vi "bg image creation-U16.vi"(0 "Array in":path[](array[path])=[path "G:/ViFFIdata/170721EuglenaN+N-/170721EuglenaN--7/N--7_00001.tif", path "G:/ViFFIdata/170721EuglenaN+N-/170721EuglenaN--7/N--7_00002.tif", path "G:/ViFFIdata/170721EuglenaN+N-/170721EuglenaN--7/N--7_00003.tif", path "G:/ViFFIdata/170721EuglenaN+N-/170721EuglenaN--7/N--7_00004.tif", path "G:/ViFFIdata/170721EuglenaN+N-/170721EuglenaN--7/N--7_00005.tif", path "G:/ViFFIdata/170721EuglenaN+N-/170721EuglenaN--7/N--7_00006.tif", path "G:/ViFFIdata/170721EuglenaN+N-/170721EuglenaN--7/N--7_00007.tif", path "G:/ViFFIdata/170721EuglenaN+N-/170721EuglenaN--7/N--7_00008.tif", path "G:/ViFFIdata/170721EuglenaN+N-/170721EuglenaN--7/N--7_00009.tif", path "G:/ViFFIdata/170721EuglenaN+N-/170721EuglenaN--7/N--7_00010.tif", path "G:/ViFFIdata/170721EuglenaN+N-/170721EuglenaN--7/N--7_00011.tif", path "G:/ViFFIdata/170721EuglenaN+N-/170721EuglenaN--7/N--7_00012.tif", path "G:/ViFFIdata/170721EuglenaN+N-/170721EuglenaN--7/N--7_00013.tif", path "G:/ViFFIdata/170721EuglenaN+N-/170721EuglenaN--7/N--7_00014.tif", path "G:/ViFFIdata/170721EuglenaN+N-/170721EuglenaN--7/N--7_00015.tif", path "G:/ViFFIdata/170721EuglenaN+N-/170721EuglenaN--7/N--7_00016.tif", path "G:/ViFFIdata/170721EuglenaN+N-/170721EuglenaN--7/N--7_00017.tif", path "G:/ViFFIdata/170721EuglenaN+N-/170721EuglenaN--7/N--7_00018.tif", path "G:/ViFFIdata/170721EuglenaN+N-/170721EuglenaN--7/N--7_00019.tif", path "G:/ViFFIdata/170721EuglenaN+N-/170721EuglenaN--7/N--7_00020.tif", path "G:/ViFFIdata/170721EuglenaN+N-/170721EuglenaN--7/N--7_00021.tif", path "G:/ViFFIdata/170721EuglenaN+N-/170721EuglenaN--7/N--7_00022.tif", path "G:/ViFFIdata/170721EuglenaN+N-/170721EuglenaN--7/N--7_00023.tif", path "G:/ViFFIdata/170721EuglenaN+N-/170721EuglenaN--7/N--7_00024.tif", path "G:/ViFFIdata/170721EuglenaN+N-/170721EuglenaN--7/N--7_00025.tif", path "G:/ViFFIdata/170721EuglenaN+N-/170721EuglenaN--7/N--7_00026.tif", path "G:/ViFFIdata/170721EuglenaN+N-/170721EuglenaN--7/N--7_00027.tif", path "G:/ViFFIdata/170721EuglenaN+N-/170721EuglenaN--7/N--7_00028.tif", path "G:/ViFFIdata/170721EuglenaN+N-/170721EuglenaN--7/N--7_00029.tif", path "G:/ViFFIdata/170721EuglenaN+N-/170721EuglenaN--7/N--7_00030.tif", path "G:/ViFFIdata/170721EuglenaN+N-/170721EuglenaN--7/N--7_00031.tif", path "G:/ViFFIdata/170721EuglenaN+N-/170721EuglenaN--7/N--7_00032.tif", path "G:/ViFFIdata/170721EuglenaN+N-/170721EuglenaN--7/N--7_00033.tif", path "G:/ViFFIdata/170721EuglenaN+N-/170721EuglenaN--7/N--7_00034.tif", path "G:/ViFFIdata/170721EuglenaN+N-/170721EuglenaN--7/N--7_00035.tif", path "G:/ViFFIdata/170721EuglenaN+N-/170721EuglenaN--7/N--7_00036.tif", path "G:/ViFFIdata/170721EuglenaN+N-/170721EuglenaN--7/N--7_00037.tif", path "G:/ViFFIdata/170721EuglenaN+N-/170721EuglenaN--7/N--7_00038.tif", path "G:/ViFFIdata/170721EuglenaN+N-/170721EuglenaN--7/N--7_00039.tif", path "G:/ViFFIdata/170721EuglenaN+N-/170721EuglenaN--7/N--7_00040.tif", path "G:/ViFFIdata/170721EuglenaN+N-/170721EuglenaN--7/N--7_00041.tif", path "G:/ViFFIdata/170721EuglenaN+N-/170721EuglenaN--7/N--7_00042.tif", path "G:/ViFFIdata/170721EuglenaN+N-/170721EuglenaN--7/N--7_00043.tif", path "G:/ViFFIdata/170721EuglenaN+N-/170721EuglenaN--7/N--7_00044.tif", path "G:/ViFFIdata/170721EuglenaN+N-/170721EuglenaN--7/N--7_00045.tif", path "G:/ViFFIdata/170721EuglenaN+N-/170721EuglenaN--7/N--7_00046.tif", path "G:/ViFFIdata/170721EuglenaN+N-/170721EuglenaN--7/N--7_00047.tif", path "G:/ViFFIdata/170721EuglenaN+N-/170721EuglenaN--7/N--7_00048.tif", path "G:/ViFFIdata/170721EuglenaN+N-/170721EuglenaN--7/N--7_00049.tif", path "G:/ViFFIdata/170721EuglenaN+N-/170721EuglenaN--7/N--7_00050.tif", path "G:/ViFFIdata/170721EuglenaN+N-/170721EuglenaN--7/N--7_00051.tif", path "G:/ViFFIdata/170721EuglenaN+N-/170721EuglenaN--7/N--7_00052.tif", path "G:/ViFFIdata/170721EuglenaN+N-/170721EuglenaN--7/N--7_00053.tif", path "G:/ViFFIdata/170721EuglenaN+N-/170721EuglenaN--7/N--7_00054.tif", path "G:/ViFFIdata/170721EuglenaN+N-/170721EuglenaN--7/N--7_00055.tif", path "G:/ViFFIdata/170721EuglenaN+N-/170721EuglenaN--7/N--7_00056.tif", path "G:/ViFFIdata/170721EuglenaN+N-/170721EuglenaN--7/N--7_00057.tif", path "G:/ViFFIdata/170721EuglenaN+N-/170721EuglenaN--7/N--7_00058.tif", path "G:/ViFFIdata/170721EuglenaN+N-/170721EuglenaN--7/N--7_00059.tif", path "G:/ViFFIdata/170721EuglenaN+N-/170721EuglenaN--7/N--7_00060.tif", path "G:/ViFFIdata/170721EuglenaN+N-/170721EuglenaN--7/N--7_00061.tif", path "G:/ViFFIdata/170721EuglenaN+N-/170721EuglenaN--7/N--7_00062.tif", path "G:/ViFFIdata/170721EuglenaN+N-/170721EuglenaN--7/N--7_00063.tif", path "G:/ViFFIdata/170721EuglenaN+N-/170721EuglenaN--7/N--7_00064.tif", path "G:/ViFFIdata/170721EuglenaN+N-/170721EuglenaN--7/N--7_00065.tif", path "G:/ViFFIdata/170721EuglenaN+N-/170721EuglenaN--7/N--7_00066.tif", path "G:/ViFFIdata/170721EuglenaN+N-/170721EuglenaN--7/N--7_00067.tif", path "G:/ViFFIdata/170721EuglenaN+N-/170721EuglenaN--7/N--7_00068.tif", path "G:/ViFFIdata/170721EuglenaN+N-/170721EuglenaN--7/N--7_00069.tif", path "G:/ViFFIdata/170721EuglenaN+N-/170721EuglenaN--7/N--7_00070.tif", path "G:/ViFFIdata/170721EuglenaN+N-/170721EuglenaN--7/N--7_00071.tif", path "G:/ViFFIdata/170721EuglenaN+N-/170721EuglenaN--7/N--7_00072.tif", path "G:/ViFFIdata/170721EuglenaN+N-/170721EuglenaN--7/N--7_00073.tif", path "G:/ViFFIdata/170721EuglenaN+N-/170721EuglenaN--7/N--7_00074.tif", path "G:/ViFFIdata/170721EuglenaN+N-/170721EuglenaN--7/N--7_00075.tif", path "G:/ViFFIdata/170721EuglenaN+N-/170721EuglenaN--7/N--7_00076.tif", path "G:/ViFFIdata/170721EuglenaN+N-/170721EuglenaN--7/N--7_00077.tif", path "G:/ViFFIdata/170721EuglenaN+N-/170721EuglenaN--7/N--7_00078.tif", path "G:/ViFFIdata/170721EuglenaN+N-/170721EuglenaN--7/N--7_00079.tif", path "G:/ViFFIdata/170721EuglenaN+N-/170721EuglenaN--7/N--7_00080.tif", path "G:/ViFFIdata/170721EuglenaN+N-/170721EuglenaN--7/N--7_00081.tif", path "G:/ViFFIdata/170721EuglenaN+N-/170721EuglenaN--7/N--7_00082.tif", path "G:/ViFFIdata/170721EuglenaN+N-/170721EuglenaN--7/N--7_00083.tif", path "G:/ViFFIdata/170721EuglenaN+N-/170721EuglenaN--7/N--7_00084.tif", path "G:/ViFFIdata/170721EuglenaN+N-/170721EuglenaN--7/N--7_00085.tif", path "G:/ViFFIdata/170721EuglenaN+N-/170721EuglenaN--7/N--7_00086.tif", path "G:/ViFFIdata/170721EuglenaN+N-/170721EuglenaN--7/N--7_00087.tif", path "G:/ViFFIdata/170721EuglenaN+N-/170721EuglenaN--7/N--7_00088.tif", path "G:/ViFFIdata/170721EuglenaN+N-/170721EuglenaN--7/N--7_00089.tif", path "G:/ViFFIdata/170721EuglenaN+N-/170721EuglenaN--7/N--7_00090.tif", path "G:/ViFFIdata/170721EuglenaN+N-/170721EuglenaN--7/N--7_00091.tif", path "G:/ViFFIdata/170721EuglenaN+N-/170721EuglenaN--7/N--7_00092.tif", path "G:/ViFFIdata/170721EuglenaN+N-/170721EuglenaN--7/N--7_00093.tif", path "G:/ViFFIdata/170721EuglenaN+N-/170721EuglenaN--7/N--7_00094.tif", path "G:/ViFFIdata/170721EuglenaN+N-/170721EuglenaN--7/N--7_00095.tif", path "G:/ViFFIdata/170721EuglenaN+N-/170721EuglenaN--7/N--7_00096.tif", path "G:/ViFFIdata/170721EuglenaN+N-/170721EuglenaN--7/N--7_00097.tif", path "G:/ViFFIdata/170721EuglenaN+N-/170721EuglenaN--7/N--7_00098.tif", path "G:/ViFFIdata/170721EuglenaN+N-/170721EuglenaN--7/N--7_00099.tif", path "G:/ViFFIdata/170721EuglenaN+N-/170721EuglenaN--7/N--7_00100.tif", path "G:/ViFFIdata/170721EuglenaN+N-/170721EuglenaN--7/N--7_00101.tif", path "G:/ViFFIdata/170721EuglenaN+N-/170721EuglenaN--7/N--7_00102.tif", path "G:/ViFFIdata/170721EuglenaN+N-/170721EuglenaN--7/N--7_00103.tif", path "G:/ViFFIdata/170721EuglenaN+N-/170721EuglenaN--7/N--7_00104.tif", path "G:/ViFFIdata/170721EuglenaN+N-/170721EuglenaN--7/N--7_00105.tif", path "G:/ViFFIdata/170721EuglenaN+N-/170721EuglenaN--7/N--7_00106.tif", path "G:/ViFFIdata/170721EuglenaN+N-/170721EuglenaN--7/N--7_00107.tif", path "G:/ViFFIdata/170721EuglenaN+N-/170721EuglenaN--7/N--7_00108.tif", path "G:/ViFFIdata/170721EuglenaN+N-/170721EuglenaN--7/N--7_00109.tif", path "G:/ViFFIdata/170721EuglenaN+N-/170721EuglenaN--7/N--7_00110.tif", path "G:/ViFFIdata/170721EuglenaN+N-/170721EuglenaN--7/N--7_00111.tif", path "G:/ViFFIdata/170721EuglenaN+N-/170721EuglenaN--7/N--7_00112.tif", path "G:/ViFFIdata/170721EuglenaN+N-/170721EuglenaN--7/N--7_00113.tif", path "G:/ViFFIdata/170721EuglenaN+N-/170721EuglenaN--7/N--7_00114.tif", path "G:/ViFFIdata/170721EuglenaN+N-/170721EuglenaN--7/N--7_00115.tif", path "G:/ViFFIdata/170721EuglenaN+N-/170721EuglenaN--7/N--7_00116.tif", path "G:/ViFFIdata/170721EuglenaN+N-/170721EuglenaN--7/N--7_00117.tif", path "G:/ViFFIdata/170721EuglenaN+N-/170721EuglenaN--7/N--7_00118.tif", path "G:/ViFFIdata/170721EuglenaN+N-/170721EuglenaN--7/N--7_00119.tif", path "G:/ViFFIdata/170721EuglenaN+N-/170721EuglenaN--7/N--7_00120.tif", path "G:/ViFFIdata/170721EuglenaN+N-/170721EuglenaN--7/N--7_00121.tif", path "G:/ViFFIdata/170721EuglenaN+N-/170721EuglenaN--7/N--7_00122.tif", path "G:/ViFFIdata/170721EuglenaN+N-/170721EuglenaN--7/N--7_00123.tif", path "G:/ViFFIdata/170721EuglenaN+N-/170721EuglenaN--7/N--7_00124.tif", path "G:/ViFFIdata/170721EuglenaN+N-/170721EuglenaN--7/N--7_00125.tif", path "G:/ViFFIdata/170721EuglenaN+N-/170721EuglenaN--7/N--7_00126.tif", path "G:/ViFFIdata/170721EuglenaN+N-/170721EuglenaN--7/N--7_00127.tif", path "G:/ViFFIdata/170721EuglenaN+N-/170721EuglenaN--7/N--7_00128.tif", path "G:/ViFFIdata/170721EuglenaN+N-/170721EuglenaN--7/N--7_00129.tif", path "G:/ViFFIdata/170721EuglenaN+N-/170721EuglenaN--7/N--7_00130.tif", path "G:/ViFFIdata/170721EuglenaN+N-/170721EuglenaN--7/N--7_00131.tif", path "G:/ViFFIdata/170721EuglenaN+N-/170721EuglenaN--7/N--7_00132.tif", path "G:/ViFFIdata/170721EuglenaN+N-/170721EuglenaN--7/N--7_00133.tif", path "G:/ViFFIdata/170721EuglenaN+N-/170721EuglenaN--7/N--7_00134.tif", path "G:/ViFFIdata/170721EuglenaN+N-/170721EuglenaN--7/N--7_00135.tif", path "G:/ViFFIdata/170721EuglenaN+N-/170721EuglenaN--7/N--7_00136.tif", path "G:/ViFFIdata/170721EuglenaN+N-/170721EuglenaN--7/N--7_00137.tif", path "G:/ViFFIdata/170721EuglenaN+N-/170721EuglenaN--7/N--7_00138.tif", path "G:/ViFFIdata/170721EuglenaN+N-/170721EuglenaN--7/N--7_00139.tif", path "G:/ViFFIdata/170721EuglenaN+N-/170721EuglenaN--7/N--7_00140.tif", path "G:/ViFFIdata/170721EuglenaN+N-/170721EuglenaN--7/N--7_00141.tif", path "G:/ViFFIdata/170721EuglenaN+N-/170721EuglenaN--7/N--7_00142.tif", path "G:/ViFFIdata/170721EuglenaN+N-/170721EuglenaN--7/N--7_00143.tif", path "G:/ViFFIdata/170721EuglenaN+N-/170721EuglenaN--7/N--7_00144.tif", path "G:/ViFFIdata/170721EuglenaN+N-/170721EuglenaN--7/N--7_00145.tif", path "G:/ViFFIdata/170721EuglenaN+N-/170721EuglenaN--7/N--7_00146.tif", path "G:/ViFFIdata/170721EuglenaN+N-/170721EuglenaN--7/N--7_00147.tif", path "G:/ViFFIdata/170721EuglenaN+N-/170721EuglenaN--7/N--7_00148.tif", path "G:/ViFFIdata/170721EuglenaN+N-/170721EuglenaN--7/N--7_00149.tif", path "G:/ViFFIdata/170721EuglenaN+N-/170721EuglenaN--7/N--7_00150.tif", path "G:/ViFFIdata/170721EuglenaN+N-/170721EuglenaN--7/N--7_00151.tif", path "G:/ViFFIdata/170721EuglenaN+N-/170721EuglenaN--7/N--7_00152.tif", path "G:/ViFFIdata/170721EuglenaN+N-/170721EuglenaN--7/N--7_00153.tif", path "G:/ViFFIdata/170721EuglenaN+N-/170721EuglenaN--7/N--7_00154.tif", path "G:/ViFFIdata/170721EuglenaN+N-/170721EuglenaN--7/N--7_00155.tif", path "G:/ViFFIdata/170721EuglenaN+N-/170721EuglenaN--7/N--7_00156.tif", path "G:/ViFFIdata/170721EuglenaN+N-/170721EuglenaN--7/N--7_00157.tif", path "G:/ViFFIdata/170721EuglenaN+N-/170721EuglenaN--7/N--7_00158.tif", path "G:/ViFFIdata/170721EuglenaN+N-/170721EuglenaN--7/N--7_00159.tif", path "G:/ViFFIdata/170721EuglenaN+N-/170721EuglenaN--7/N--7_00160.tif", path "G:/ViFFIdata/170721EuglenaN+N-/170721EuglenaN--7/N--7_00161.tif", path "G:/ViFFIdata/170721EuglenaN+N-/170721EuglenaN--7/N--7_00162.tif", path "G:/ViFFIdata/170721EuglenaN+N-/170721EuglenaN--7/N--7_00163.tif", path "G:/ViFFIdata/170721EuglenaN+N-/170721EuglenaN--7/N--7_00164.tif", path "G:/ViFFIdata/170721EuglenaN+N-/170721EuglenaN--7/N--7_00165.tif", path "G:/ViFFIdata/170721EuglenaN+N-/170721EuglenaN--7/N--7_00166.tif", path "G:/ViFFIdata/170721EuglenaN+N-/170721EuglenaN--7/N--7_00167.tif", path "G:/ViFFIdata/170721EuglenaN+N-/170721EuglenaN--7/N--7_00168.tif", path "G:/ViFFIdata/170721EuglenaN+N-/170721EuglenaN--7/N--7_00169.tif", path "G:/ViFFIdata/170721EuglenaN+N-/170721EuglenaN--7/N--7_00170.tif", path "G:/ViFFIdata/170721EuglenaN+N-/170721EuglenaN--7/N--7_00171.tif", path "G:/ViFFIdata/170721EuglenaN+N-/170721EuglenaN--7/N--7_00172.tif", path "G:/ViFFIdata/170721EuglenaN+N-/170721EuglenaN--7/N--7_00173.tif", path "G:/ViFFIdata/170721EuglenaN+N-/170721EuglenaN--7/N--7_00174.tif", path "G:/ViFFIdata/170721EuglenaN+N-/170721EuglenaN--7/N--7_00175.tif", path "G:/ViFFIdata/170721EuglenaN+N-/170721EuglenaN--7/N--7_00176.tif", path "G:/ViFFIdata/170721EuglenaN+N-/170721EuglenaN--7/N--7_00177.tif", path "G:/ViFFIdata/170721EuglenaN+N-/170721EuglenaN--7/N--7_00178.tif", path "G:/ViFFIdata/170721EuglenaN+N-/170721EuglenaN--7/N--7_00179.tif", path "G:/ViFFIdata/170721EuglenaN+N-/170721EuglenaN--7/N--7_00180.tif", path "G:/ViFFIdata/170721EuglenaN+N-/170721EuglenaN--7/N--7_00181.tif", path "G:/ViFFIdata/170721EuglenaN+N-/170721EuglenaN--7/N--7_00182.tif", path "G:/ViFFIdata/170721EuglenaN+N-/170721EuglenaN--7/N--7_00183.tif", path "G:/ViFFIdata/170721EuglenaN+N-/170721EuglenaN--7/N--7_00184.tif", path "G:/ViFFIdata/170721EuglenaN+N-/170721EuglenaN--7/N--7_00185.tif", path "G:/ViFFIdata/170721EuglenaN+N-/170721EuglenaN--7/N--7_00186.tif", path "G:/ViFFIdata/170721EuglenaN+N-/170721EuglenaN--7/N--7_00187.tif", path "G:/ViFFIdata/170721EuglenaN+N-/170721EuglenaN--7/N--7_00188.tif", path "G:/ViFFIdata/170721EuglenaN+N-/170721EuglenaN--7/N--7_00189.tif", path "G:/ViFFIdata/170721EuglenaN+N-/170721EuglenaN--7/N--7_00190.tif", path "G:/ViFFIdata/170721EuglenaN+N-/170721EuglenaN--7/N--7_00191.tif", path "G:/ViFFIdata/170721EuglenaN+N-/170721EuglenaN--7/N--7_00192.tif", path "G:/ViFFIdata/170721EuglenaN+N-/170721EuglenaN--7/N--7_00193.tif", path "G:/ViFFIdata/170721EuglenaN+N-/170721EuglenaN--7/N--7_00194.tif", path "G:/ViFFIdata/170721EuglenaN+N-/170721EuglenaN--7/N--7_00195.tif", path "G:/ViFFIdata/170721EuglenaN+N-/170721EuglenaN--7/N--7_00196.tif", path "G:/ViFFIdata/170721EuglenaN+N-/170721EuglenaN--7/N--7_00197.tif", path "G:/ViFFIdata/170721EuglenaN+N-/170721EuglenaN--7/N--7_00198.tif", path "G:/ViFFIdata/170721EuglenaN+N-/170721EuglenaN--7/N--7_00199.tif", path "G:/ViFFIdata/170721EuglenaN+N-/170721EuglenaN--7/N--7_00200.tif", path "G:/ViFFIdata/170721EuglenaN+N-/170721EuglenaN--7/N--7_00201.tif", path "G:/ViFFIdata/170721EuglenaN+N-/170721EuglenaN--7/N--7_00202.tif", path "G:/ViFFIdata/170721EuglenaN+N-/170721EuglenaN--7/N--7_00203.tif", path "G:/ViFFIdata/170721EuglenaN+N-/170721EuglenaN--7/N--7_00204.tif", path "G:/ViFFIdata/170721EuglenaN+N-/170721EuglenaN--7/N--7_00205.tif", path "G:/ViFFIdata/170721EuglenaN+N-/170721EuglenaN--7/N--7_00206.tif", path "G:/ViFFIdata/170721EuglenaN+N-/170721EuglenaN--7/N--7_00207.tif", path "G:/ViFFIdata/170721EuglenaN+N-/170721EuglenaN--7/N--7_00208.tif", path "G:/ViFFIdata/170721EuglenaN+N-/170721EuglenaN--7/N--7_00209.tif", path "G:/ViFFIdata/170721EuglenaN+N-/170721EuglenaN--7/N--7_00210.tif", path "G:/ViFFIdata/170721EuglenaN+N-/170721EuglenaN--7/N--7_00211.tif", path "G:/ViFFIdata/170721EuglenaN+N-/170721EuglenaN--7/N--7_00212.tif", path "G:/ViFFIdata/170721EuglenaN+N-/170721EuglenaN--7/N--7_00213.tif", path "G:/ViFFIdata/170721EuglenaN+N-/170721EuglenaN--7/N--7_00214.tif", path "G:/ViFFIdata/170721EuglenaN+N-/170721EuglenaN--7/N--7_00215.tif", path "G:/ViFFIdata/170721EuglenaN+N-/170721EuglenaN--7/N--7_00216.tif", path "G:/ViFFIdata/170721EuglenaN+N-/170721EuglenaN--7/N--7_00217.tif", path "G:/ViFFIdata/170721EuglenaN+N-/170721EuglenaN--7/N--7_00218.tif", path "G:/ViFFIdata/170721EuglenaN+N-/170721EuglenaN--7/N--7_00219.tif", path "G:/ViFFIdata/170721EuglenaN+N-/170721EuglenaN--7/N--7_00220.tif", path "G:/ViFFIdata/170721EuglenaN+N-/170721EuglenaN--7/N--7_00221.tif", path "G:/ViFFIdata/170721EuglenaN+N-/170721EuglenaN--7/N--7_00222.tif", path "G:/ViFFIdata/170721EuglenaN+N-/170721EuglenaN--7/N--7_00223.tif", path "G:/ViFFIdata/170721EuglenaN+N-/170721EuglenaN--7/N--7_00224.tif", path "G:/ViFFIdata/170721EuglenaN+N-/170721EuglenaN--7/N--7_00225.tif", path "G:/ViFFIdata/170721EuglenaN+N-/170721EuglenaN--7/N--7_00226.tif", path "G:/ViFFIdata/170721EuglenaN+N-/170721EuglenaN--7/N--7_00227.tif", path "G:/ViFFIdata/170721EuglenaN+N-/170721EuglenaN--7/N--7_00228.tif", path "G:/ViFFIdata/170721EuglenaN+N-/170721EuglenaN--7/N--7_00229.tif", path "G:/ViFFIdata/170721EuglenaN+N-/170721EuglenaN--7/N--7_00230.tif", path "G:/ViFFIdata/170721EuglenaN+N-/170721EuglenaN--7/N--7_00231.tif", path "G:/ViFFIdata/170721EuglenaN+N-/170721EuglenaN--7/N--7_00232.tif", path "G:/ViFFIdata/170721EuglenaN+N-/170721EuglenaN--7/N--7_00233.tif", path "G:/ViFFIdata/170721EuglenaN+N-/170721EuglenaN--7/N--7_00234.tif", path "G:/ViFFIdata/170721EuglenaN+N-/170721EuglenaN--7/N--7_00235.tif", path "G:/ViFFIdata/170721EuglenaN+N-/170721EuglenaN--7/N--7_00236.tif", path "G:/ViFFIdata/170721EuglenaN+N-/170721EuglenaN--7/N--7_00237.tif", path "G:/ViFFIdata/170721EuglenaN+N-/170721EuglenaN--7/N--7_00238.tif", path "G:/ViFFIdata/170721EuglenaN+N-/170721EuglenaN--7/N--7_00239.tif", path "G:/ViFFIdata/170721EuglenaN+N-/170721EuglenaN--7/N--7_00240.tif", path "G:/ViFFIdata/170721EuglenaN+N-/170721EuglenaN--7/N--7_00241.tif", path "G:/ViFFIdata/170721EuglenaN+N-/170721EuglenaN--7/N--7_00242.tif", path "G:/ViFFIdata/170721EuglenaN+N-/170721EuglenaN--7/N--7_00243.tif", path "G:/ViFFIdata/170721EuglenaN+N-/170721EuglenaN--7/N--7_00244.tif", path "G:/ViFFIdata/170721EuglenaN+N-/170721EuglenaN--7/N--7_00245.tif", path "G:/ViFFIdata/170721EuglenaN+N-/170721EuglenaN--7/N--7_00246.tif", path "G:/ViFFIdata/170721EuglenaN+N-/170721EuglenaN--7/N--7_00247.tif", path "G:/ViFFIdata/170721EuglenaN+N-/170721EuglenaN--7/N--7_00248.tif", path "G:/ViFFIdata/170721EuglenaN+N-/170721EuglenaN--7/N--7_00249.tif", path "G:/ViFFIdata/170721EuglenaN+N-/170721EuglenaN--7/N--7_00250.tif", path "G:/ViFFIdata/170721EuglenaN+N-/170721EuglenaN--7/N--7_00251.tif", path "G:/ViFFIdata/170721EuglenaN+N-/170721EuglenaN--7/N--7_00252.tif", path "G:/ViFFIdata/170721EuglenaN+N-/170721EuglenaN--7/N--7_00253.tif", path "G:/ViFFIdata/170721EuglenaN+N-/170721EuglenaN--7/N--7_00254.tif", path "G:/ViFFIdata/170721EuglenaN+N-/170721EuglenaN--7/N--7_00255.tif", path "G:/ViFFIdata/170721EuglenaN+N-/170721EuglenaN--7/N--7_00256.tif", path "G:/ViFFIdata/170721EuglenaN+N-/170721EuglenaN--7/N--7_00257.tif", path "G:/ViFFIdata/170721EuglenaN+N-/170721EuglenaN--7/N--7_00258.tif", path "G:/ViFFIdata/170721EuglenaN+N-/170721EuglenaN--7/N--7_00259.tif", path "G:/ViFFIdata/170721EuglenaN+N-/170721EuglenaN--7/N--7_00260.tif", path "G:/ViFFIdata/170721EuglenaN+N-/170721EuglenaN--7/N--7_00261.tif", path "G:/ViFFIdata/170721EuglenaN+N-/170721EuglenaN--7/N--7_00262.tif", path "G:/ViFFIdata/170721EuglenaN+N-/170721EuglenaN--7/N--7_00263.tif", path "G:/ViFFIdata/170721EuglenaN+N-/170721EuglenaN--7/N--7_00264.tif", path "G:/ViFFIdata/170721EuglenaN+N-/170721EuglenaN--7/N--7_00265.tif", path "G:/ViFFIdata/170721EuglenaN+N-/170721EuglenaN--7/N--7_00266.tif", path "G:/ViFFIdata/170721EuglenaN+N-/170721EuglenaN--7/N--7_00267.tif", path "G:/ViFFIdata/170721EuglenaN+N-/170721EuglenaN--7/N--7_00268.tif", path "G:/ViFFIdata/170721EuglenaN+N-/170721EuglenaN--7/N--7_00269.tif", path "G:/ViFFIdata/170721EuglenaN+N-/170721EuglenaN--7/N--7_00270.tif", path "G:/ViFFIdata/170721EuglenaN+N-/170721EuglenaN--7/N--7_00271.tif", path "G:/ViFFIdata/170721EuglenaN+N-/170721EuglenaN--7/N--7_00272.tif", path "G:/ViFFIdata/170721EuglenaN+N-/170721EuglenaN--7/N--7_00273.tif", path "G:/ViFFIdata/170721EuglenaN+N-/170721EuglenaN--7/N--7_00274.tif", path "G:/ViFFIdata/170721EuglenaN+N-/170721EuglenaN--7/N--7_00275.tif", path "G:/ViFFIdata/170721EuglenaN+N-/170721EuglenaN--7/N--7_00276.tif", path "G:/ViFFIdata/170721EuglenaN+N-/170721EuglenaN--7/N--7_00277.tif", path "G:/ViFFIdata/170721EuglenaN+N-/170721EuglenaN--7/N--7_00278.tif", path "G:/ViFFIdata/170721EuglenaN+N-/170721EuglenaN--7/N--7_00279.tif", path "G:/ViFFIdata/170721EuglenaN+N-/170721EuglenaN--7/N--7_00280.tif", path "G:/ViFFIdata/170721EuglenaN+N-/170721EuglenaN--7/N--7_00281.tif", path "G:/ViFFIdata/170721EuglenaN+N-/170721EuglenaN--7/N--7_00282.tif", path "G:/ViFFIdata/170721EuglenaN+N-/170721EuglenaN--7/N--7_00283.tif", path "G:/ViFFIdata/170721EuglenaN+N-/170721EuglenaN--7/N--7_00284.tif", path "G:/ViFFIdata/170721EuglenaN+N-/170721EuglenaN--7/N--7_00285.tif", path "G:/ViFFIdata/170721EuglenaN+N-/170721EuglenaN--7/N--7_00286.tif", path "G:/ViFFIdata/170721EuglenaN+N-/170721EuglenaN--7/N--7_00287.tif", path "G:/ViFFIdata/170721EuglenaN+N-/170721EuglenaN--7/N--7_00288.tif", path "G:/ViFFIdata/170721EuglenaN+N-/170721EuglenaN--7/N--7_00289.tif", path "G:/ViFFIdata/170721EuglenaN+N-/170721EuglenaN--7/N--7_00290.tif", path "G:/ViFFIdata/170721EuglenaN+N-/170721EuglenaN--7/N--7_00291.tif", path "G:/ViFFIdata/170721EuglenaN+N-/170721EuglenaN--7/N--7_00292.tif", path "G:/ViFFIdata/170721EuglenaN+N-/170721EuglenaN--7/N--7_00293.tif", path "G:/ViFFIdata/170721EuglenaN+N-/170721EuglenaN--7/N--7_00294.tif", path "G:/ViFFIdata/170721EuglenaN+N-/170721EuglenaN--7/N--7_00295.tif", path "G:/ViFFIdata/170721EuglenaN+N-/170721EuglenaN--7/N--7_00296.tif", path "G:/ViFFIdata/170721EuglenaN+N-/170721EuglenaN--7/N--7_00297.tif", path "G:/ViFFIdata/170721EuglenaN+N-/170721EuglenaN--7/N--7_00298.tif", path "G:/ViFFIdata/170721EuglenaN+N-/170721EuglenaN--7/N--7_00299.tif", path "G:/ViFFIdata/170721EuglenaN+N-/170721EuglenaN--7/N--7_00300.tif", path "G:/ViFFIdata/170721EuglenaN+N-/170721EuglenaN--7/N--7_00301.tif", path "G:/ViFFIdata/170721EuglenaN+N-/170721EuglenaN--7/N--7_00302.tif", path "G:/ViFFIdata/170721EuglenaN+N-/170721EuglenaN--7/N--7_00303.tif", path "G:/ViFFIdata/170721EuglenaN+N-/170721EuglenaN--7/N--7_00304.tif", path "G:/ViFFIdata/170721EuglenaN+N-/170721EuglenaN--7/N--7_00305.tif", path "G:/ViFFIdata/170721EuglenaN+N-/170721EuglenaN--7/N--7_00306.tif", path "G:/ViFFIdata/170721EuglenaN+N-/170721EuglenaN--7/N--7_00307.tif", path "G:/ViFFIdata/170721EuglenaN+N-/170721EuglenaN--7/N--7_00308.tif", path "G:/ViFFIdata/170721EuglenaN+N-/170721EuglenaN--7/N--7_00309.tif", path "G:/ViFFIdata/170721EuglenaN+N-/170721EuglenaN--7/N--7_00310.tif", path "G:/ViFFIdata/170721EuglenaN+N-/170721EuglenaN--7/N--7_00311.tif", path "G:/ViFFIdata/170721EuglenaN+N-/170721EuglenaN--7/N--7_00312.tif", path "G:/ViFFIdata/170721EuglenaN+N-/170721EuglenaN--7/N--7_00313.tif", path "G:/ViFFIdata/170721EuglenaN+N-/170721EuglenaN--7/N--7_00314.tif", path "G:/ViFFIdata/170721EuglenaN+N-/170721EuglenaN--7/N--7_00315.tif", path "G:/ViFFIdata/170721EuglenaN+N-/170721EuglenaN--7/N--7_00316.tif", path "G:/ViFFIdata/170721EuglenaN+N-/170721EuglenaN--7/N--7_00317.tif", path "G:/ViFFIdata/170721EuglenaN+N-/170721EuglenaN--7/N--7_00318.tif", path "G:/ViFFIdata/170721EuglenaN+N-/170721EuglenaN--7/N--7_00319.tif", path "G:/ViFFIdata/170721EuglenaN+N-/170721EuglenaN--7/N--7_00320.tif", path "G:/ViFFIdata/170721EuglenaN+N-/170721EuglenaN--7/N--7_00321.tif", path "G:/ViFFIdata/170721EuglenaN+N-/170721EuglenaN--7/N--7_00322.tif", path "G:/ViFFIdata/170721EuglenaN+N-/170721EuglenaN--7/N--7_00323.tif", path "G:/ViFFIdata/170721EuglenaN+N-/170721EuglenaN--7/N--7_00324.tif", path "G:/ViFFIdata/170721EuglenaN+N-/170721EuglenaN--7/N--7_00325.tif", path "G:/ViFFIdata/170721EuglenaN+N-/170721EuglenaN--7/N--7_00326.tif", path "G:/ViFFIdata/170721EuglenaN+N-/170721EuglenaN--7/N--7_00327.tif", path "G:/ViFFIdata/170721EuglenaN+N-/170721EuglenaN--7/N--7_00328.tif", path "G:/ViFFIdata/170721EuglenaN+N-/170721EuglenaN--7/N--7_00329.tif", path "G:/ViFFIdata/170721EuglenaN+N-/170721EuglenaN--7/N--7_00330.tif", path "G:/ViFFIdata/170721EuglenaN+N-/170721EuglenaN--7/N--7_00331.tif", path "G:/ViFFIdata/170721EuglenaN+N-/170721EuglenaN--7/N--7_00332.tif", path "G:/ViFFIdata/170721EuglenaN+N-/170721EuglenaN--7/N--7_00333.tif", path "G:/ViFFIdata/170721EuglenaN+N-/170721EuglenaN--7/N--7_00334.tif", path "G:/ViFFIdata/170721EuglenaN+N-/170721EuglenaN--7/N--7_00335.tif", path "G:/ViFFIdata/170721EuglenaN+N-/170721EuglenaN--7/N--7_00336.tif", path "G:/ViFFIdata/170721EuglenaN+N-/170721EuglenaN--7/N--7_00337.tif", path "G:/ViFFIdata/170721EuglenaN+N-/170721EuglenaN--7/N--7_00338.tif", path "G:/ViFFIdata/170721EuglenaN+N-/170721EuglenaN--7/N--7_00339.tif", path "G:/ViFFIdata/170721EuglenaN+N-/170721EuglenaN--7/N--7_00340.tif", path "G:/ViFFIdata/170721EuglenaN+N-/170721EuglenaN--7/N--7_00341.tif", path "G:/ViFFIdata/170721EuglenaN+N-/170721EuglenaN--7/N--7_00342.tif", path "G:/ViFFIdata/170721EuglenaN+N-/170721EuglenaN--7/N--7_00343.tif", path "G:/ViFFIdata/170721EuglenaN+N-/170721EuglenaN--7/N--7_00344.tif", path "G:/ViFFIdata/170721EuglenaN+N-/170721EuglenaN--7/N--7_00345.tif", path "G:/ViFFIdata/170721EuglenaN+N-/170721EuglenaN--7/N--7_00346.tif", path "G:/ViFFIdata/170721EuglenaN+N-/170721EuglenaN--7/N--7_00347.tif", path "G:/ViFFIdata/170721EuglenaN+N-/170721EuglenaN--7/N--7_00348.tif", path "G:/ViFFIdata/170721EuglenaN+N-/170721EuglenaN--7/N--7_00349.tif", path "G:/ViFFIdata/170721EuglenaN+N-/170721EuglenaN--7/N--7_00350.tif", path "G:/ViFFIdata/170721EuglenaN+N-/170721EuglenaN--7/N--7_00351.tif", path "G:/ViFFIdata/170721EuglenaN+N-/170721EuglenaN--7/N--7_00352.tif", path "G:/ViFFIdata/170721EuglenaN+N-/170721EuglenaN--7/N--7_00353.tif", path "G:/ViFFIdata/170721EuglenaN+N-/170721EuglenaN--7/N--7_00354.tif", path "G:/ViFFIdata/170721EuglenaN+N-/170721EuglenaN--7/N--7_00355.tif", path "G:/ViFFIdata/170721EuglenaN+N-/170721EuglenaN--7/N--7_00356.tif", path "G:/ViFFIdata/170721EuglenaN+N-/170721EuglenaN--7/N--7_00357.tif", path "G:/ViFFIdata/170721EuglenaN+N-/170721EuglenaN--7/N--7_00358.tif", path "G:/ViFFIdata/170721EuglenaN+N-/170721EuglenaN--7/N--7_00359.tif", path "G:/ViFFIdata/170721EuglenaN+N-/170721EuglenaN--7/N--7_00360.tif", path "G:/ViFFIdata/170721EuglenaN+N-/170721EuglenaN--7/N--7_00361.tif", path "G:/ViFFIdata/170721EuglenaN+N-/170721EuglenaN--7/N--7_00362.tif", path "G:/ViFFIdata/170721EuglenaN+N-/170721EuglenaN--7/N--7_00363.tif", path "G:/ViFFIdata/170721EuglenaN+N-/170721EuglenaN--7/N--7_00364.tif", path "G:/ViFFIdata/170721EuglenaN+N-/170721EuglenaN--7/N--7_00365.tif", path "G:/ViFFIdata/170721EuglenaN+N-/170721EuglenaN--7/N--7_00366.tif", path "G:/ViFFIdata/170721EuglenaN+N-/170721EuglenaN--7/N--7_00367.tif", path "G:/ViFFIdata/170721EuglenaN+N-/170721EuglenaN--7/N--7_00368.tif", path "G:/ViFFIdata/170721EuglenaN+N-/170721EuglenaN--7/N--7_00369.tif", path "G:/ViFFIdata/170721EuglenaN+N-/170721EuglenaN--7/N--7_00370.tif", path "G:/ViFFIdata/170721EuglenaN+N-/170721EuglenaN--7/N--7_00371.tif", path "G:/ViFFIdata/170721EuglenaN+N-/170721EuglenaN--7/N--7_00372.tif", path "G:/ViFFIdata/170721EuglenaN+N-/170721EuglenaN--7/N--7_00373.tif", path "G:/ViFFIdata/170721EuglenaN+N-/170721EuglenaN--7/N--7_00374.tif", path "G:/ViFFIdata/170721EuglenaN+N-/170721EuglenaN--7/N--7_00375.tif", path "G:/ViFFIdata/170721EuglenaN+N-/170721EuglenaN--7/N--7_00376.tif", path "G:/ViFFIdata/170721EuglenaN+N-/170721EuglenaN--7/N--7_00377.tif", path "G:/ViFFIdata/170721EuglenaN+N-/170721EuglenaN--7/N--7_00378.tif", path "G:/ViFFIdata/170721EuglenaN+N-/170721EuglenaN--7/N--7_00379.tif", path "G:/ViFFIdata/170721EuglenaN+N-/170721EuglenaN--7/N--7_00380.tif", path "G:/ViFFIdata/170721EuglenaN+N-/170721EuglenaN--7/N--7_00381.tif", path "G:/ViFFIdata/170721EuglenaN+N-/170721EuglenaN--7/N--7_00382.tif", path "G:/ViFFIdata/170721EuglenaN+N-/170721EuglenaN--7/N--7_00383.tif", path "G:/ViFFIdata/170721EuglenaN+N-/170721EuglenaN--7/N--7_00384.tif", path "G:/ViFFIdata/170721EuglenaN+N-/170721EuglenaN--7/N--7_00385.tif", path "G:/ViFFIdata/170721EuglenaN+N-/170721EuglenaN--7/N--7_00386.tif", path "G:/ViFFIdata/170721EuglenaN+N-/170721EuglenaN--7/N--7_00387.tif", path "G:/ViFFIdata/170721EuglenaN+N-/170721EuglenaN--7/N--7_00388.tif", path "G:/ViFFIdata/170721EuglenaN+N-/170721EuglenaN--7/N--7_00389.tif", path "G:/ViFFIdata/170721EuglenaN+N-/170721EuglenaN--7/N--7_00390.tif", path "G:/ViFFIdata/170721EuglenaN+N-/170721EuglenaN--7/N--7_00391.tif", path "G:/ViFFIdata/170721EuglenaN+N-/170721EuglenaN--7/N--7_00392.tif", path "G:/ViFFIdata/170721EuglenaN+N-/170721EuglenaN--7/N--7_00393.tif", path "G:/ViFFIdata/170721EuglenaN+N-/170721EuglenaN--7/N--7_00394.tif", path "G:/ViFFIdata/170721EuglenaN+N-/170721EuglenaN--7/N--7_00395.tif", path "G:/ViFFIdata/170721EuglenaN+N-/170721EuglenaN--7/N--7_00396.tif", path "G:/ViFFIdata/170721EuglenaN+N-/170721EuglenaN--7/N--7_00397.tif", path "G:/ViFFIdata/170721EuglenaN+N-/170721EuglenaN--7/N--7_00398.tif", path "G:/ViFFIdata/170721EuglenaN+N-/170721EuglenaN--7/N--7_00399.tif", path "G:/ViFFIdata/170721EuglenaN+N-/170721EuglenaN--7/N--7_00400.tif", path "G:/ViFFIdata/170721EuglenaN+N-/170721EuglenaN--7/N--7_00401.tif", path "G:/ViFFIdata/170721EuglenaN+N-/170721EuglenaN--7/N--7_00402.tif", path "G:/ViFFIdata/170721EuglenaN+N-/170721EuglenaN--7/N--7_00403.tif", path "G:/ViFFIdata/170721EuglenaN+N-/170721EuglenaN--7/N--7_00404.tif", path "G:/ViFFIdata/170721EuglenaN+N-/170721EuglenaN--7/N--7_00405.tif", path "G:/ViFFIdata/170721EuglenaN+N-/170721EuglenaN--7/N--7_00406.tif", path "G:/ViFFIdata/170721EuglenaN+N-/170721EuglenaN--7/N--7_00407.tif", path "G:/ViFFIdata/170721EuglenaN+N-/170721EuglenaN--7/N--7_00408.tif", path "G:/ViFFIdata/170721EuglenaN+N-/170721EuglenaN--7/N--7_00409.tif", path "G:/ViFFIdata/170721EuglenaN+N-/170721EuglenaN--7/N--7_00410.tif", path "G:/ViFFIdata/170721EuglenaN+N-/170721EuglenaN--7/N--7_00411.tif", path "G:/ViFFIdata/170721EuglenaN+N-/170721EuglenaN--7/N--7_00412.tif", path "G:/ViFFIdata/170721EuglenaN+N-/170721EuglenaN--7/N--7_00413.tif", path "G:/ViFFIdata/170721EuglenaN+N-/170721EuglenaN--7/N--7_00414.tif", path "G:/ViFFIdata/170721EuglenaN+N-/170721EuglenaN--7/N--7_00415.tif", path "G:/ViFFIdata/170721EuglenaN+N-/170721EuglenaN--7/N--7_00416.tif", path "G:/ViFFIdata/170721EuglenaN+N-/170721EuglenaN--7/N--7_00417.tif", path "G:/ViFFIdata/170721EuglenaN+N-/170721EuglenaN--7/N--7_00418.tif", path "G:/ViFFIdata/170721EuglenaN+N-/170721EuglenaN--7/N--7_00419.tif", path "G:/ViFFIdata/170721EuglenaN+N-/170721EuglenaN--7/N--7_00420.tif", path "G:/ViFFIdata/170721EuglenaN+N-/170721EuglenaN--7/N--7_00421.tif", path "G:/ViFFIdata/170721EuglenaN+N-/170721EuglenaN--7/N--7_00422.tif", path "G:/ViFFIdata/170721EuglenaN+N-/170721EuglenaN--7/N--7_00423.tif", path "G:/ViFFIdata/170721EuglenaN+N-/170721EuglenaN--7/N--7_00424.tif", path "G:/ViFFIdata/170721EuglenaN+N-/170721EuglenaN--7/N--7_00425.tif", path "G:/ViFFIdata/170721EuglenaN+N-/170721EuglenaN--7/N--7_00426.tif", path "G:/ViFFIdata/170721EuglenaN+N-/170721EuglenaN--7/N--7_00427.tif", path "G:/ViFFIdata/170721EuglenaN+N-/170721EuglenaN--7/N--7_00428.tif", path "G:/ViFFIdata/170721EuglenaN+N-/170721EuglenaN--7/N--7_00429.tif", path "G:/ViFFIdata/170721EuglenaN+N-/170721EuglenaN--7/N--7_00430.tif", path "G:/ViFFIdata/170721EuglenaN+N-/170721EuglenaN--7/N--7_00431.tif", path "G:/ViFFIdata/170721EuglenaN+N-/170721EuglenaN--7/N--7_00432.tif", path "G:/ViFFIdata/170721EuglenaN+N-/170721EuglenaN--7/N--7_00433.tif", path "G:/ViFFIdata/170721EuglenaN+N-/170721EuglenaN--7/N--7_00434.tif", path "G:/ViFFIdata/170721EuglenaN+N-/170721EuglenaN--7/N--7_00435.tif", path "G:/ViFFIdata/170721EuglenaN+N-/170721EuglenaN--7/N--7_00436.tif", path "G:/ViFFIdata/170721EuglenaN+N-/170721EuglenaN--7/N--7_00437.tif", path "G:/ViFFIdata/170721EuglenaN+N-/170721EuglenaN--7/N--7_00438.tif", path "G:/ViFFIdata/170721EuglenaN+N-/170721EuglenaN--7/N--7_00439.tif", path "G:/ViFFIdata/170721EuglenaN+N-/170721EuglenaN--7/N--7_00440.tif", path "G:/ViFFIdata/170721EuglenaN+N-/170721EuglenaN--7/N--7_00441.tif", path "G:/ViFFIdata/170721EuglenaN+N-/170721EuglenaN--7/N--7_00442.tif", path "G:/ViFFIdata/170721EuglenaN+N-/170721EuglenaN--7/N--7_00443.tif", path "G:/ViFFIdata/170721EuglenaN+N-/170721EuglenaN--7/N--7_00444.tif", path "G:/ViFFIdata/170721EuglenaN+N-/170721EuglenaN--7/N--7_00445.tif", path "G:/ViFFIdata/170721EuglenaN+N-/170721EuglenaN--7/N--7_00446.tif", path "G:/ViFFIdata/170721EuglenaN+N-/170721EuglenaN--7/N--7_00447.tif", path "G:/ViFFIdata/170721EuglenaN+N-/170721EuglenaN--7/N--7_00448.tif", path "G:/ViFFIdata/170721EuglenaN+N-/170721EuglenaN--7/N--7_00449.tif", path "G:/ViFFIdata/170721EuglenaN+N-/170721EuglenaN--7/N--7_00450.tif", path "G:/ViFFIdata/170721EuglenaN+N-/170721EuglenaN--7/N--7_00451.tif", path "G:/ViFFIdata/170721EuglenaN+N-/170721EuglenaN--7/N--7_00452.tif", path "G:/ViFFIdata/170721EuglenaN+N-/170721EuglenaN--7/N--7_00453.tif", path "G:/ViFFIdata/170721EuglenaN+N-/170721EuglenaN--7/N--7_00454.tif", path "G:/ViFFIdata/170721EuglenaN+N-/170721EuglenaN--7/N--7_00455.tif", path "G:/ViFFIdata/170721EuglenaN+N-/170721EuglenaN--7/N--7_00456.tif", path "G:/ViFFIdata/170721EuglenaN+N-/170721EuglenaN--7/N--7_00457.tif", path "G:/ViFFIdata/170721EuglenaN+N-/170721EuglenaN--7/N--7_00458.tif", path "G:/ViFFIdata/170721EuglenaN+N-/170721EuglenaN--7/N--7_00459.tif", path "G:/ViFFIdata/170721EuglenaN+N-/170721EuglenaN--7/N--7_00460.tif", path "G:/ViFFIdata/170721EuglenaN+N-/170721EuglenaN--7/N--7_00461.tif", path "G:/ViFFIdata/170721EuglenaN+N-/170721EuglenaN--7/N--7_00462.tif", path "G:/ViFFIdata/170721EuglenaN+N-/170721EuglenaN--7/N--7_00463.tif", path "G:/ViFFIdata/170721EuglenaN+N-/170721EuglenaN--7/N--7_00464.tif", path "G:/ViFFIdata/170721EuglenaN+N-/170721EuglenaN--7/N--7_00465.tif", path "G:/ViFFIdata/170721EuglenaN+N-/170721EuglenaN--7/N--7_00466.tif", path "G:/ViFFIdata/170721EuglenaN+N-/170721EuglenaN--7/N--7_00467.tif", path "G:/ViFFIdata/170721EuglenaN+N-/170721EuglenaN--7/N--7_00468.tif", path "G:/ViFFIdata/170721EuglenaN+N-/170721EuglenaN--7/N--7_00469.tif", path "G:/ViFFIdata/170721EuglenaN+N-/170721EuglenaN--7/N--7_00470.tif", path "G:/ViFFIdata/170721EuglenaN+N-/170721EuglenaN--7/N--7_00471.tif", path "G:/ViFFIdata/170721EuglenaN+N-/170721EuglenaN--7/N--7_00472.tif", path "G:/ViFFIdata/170721EuglenaN+N-/170721EuglenaN--7/N--7_00473.tif", path "G:/ViFFIdata/170721EuglenaN+N-/170721EuglenaN--7/N--7_00474.tif", path "G:/ViFFIdata/170721EuglenaN+N-/170721EuglenaN--7/N--7_00475.tif", path "G:/ViFFIdata/170721EuglenaN+N-/170721EuglenaN--7/N--7_00476.tif", path "G:/ViFFIdata/170721EuglenaN+N-/170721EuglenaN--7/N--7_00477.tif", path "G:/ViFFIdata/170721EuglenaN+N-/170721EuglenaN--7/N--7_00478.tif", path "G:/ViFFIdata/170721EuglenaN+N-/170721EuglenaN--7/N--7_00479.tif", path "G:/ViFFIdata/170721EuglenaN+N-/170721EuglenaN--7/N--7_00480.tif", path "G:/ViFFIdata/170721EuglenaN+N-/170721EuglenaN--7/N--7_00481.tif", path "G:/ViFFIdata/170721EuglenaN+N-/170721EuglenaN--7/N--7_00482.tif", path "G:/ViFFIdata/170721EuglenaN+N-/170721EuglenaN--7/N--7_00483.tif", path "G:/ViFFIdata/170721EuglenaN+N-/170721EuglenaN--7/N--7_00484.tif", path "G:/ViFFIdata/170721EuglenaN+N-/170721EuglenaN--7/N--7_00485.tif", path "G:/ViFFIdata/170721EuglenaN+N-/170721EuglenaN--7/N--7_00486.tif", path "G:/ViFFIdata/170721EuglenaN+N-/170721EuglenaN--7/N--7_00487.tif", path "G:/ViFFIdata/170721EuglenaN+N-/170721EuglenaN--7/N--7_00488.tif", path "G:/ViFFIdata/170721EuglenaN+N-/170721EuglenaN--7/N--7_00489.tif", path "G:/ViFFIdata/170721EuglenaN+N-/170721EuglenaN--7/N--7_00490.tif", path "G:/ViFFIdata/170721EuglenaN+N-/170721EuglenaN--7/N--7_00491.tif", path "G:/ViFFIdata/170721EuglenaN+N-/170721EuglenaN--7/N--7_00492.tif", path "G:/ViFFIdata/170721EuglenaN+N-/170721EuglenaN--7/N--7_00493.tif", path "G:/ViFFIdata/170721EuglenaN+N-/170721EuglenaN--7/N--7_00494.tif", path "G:/ViFFIdata/170721EuglenaN+N-/170721EuglenaN--7/N--7_00495.tif", path "G:/ViFFIdata/170721EuglenaN+N-/170721EuglenaN--7/N--7_00496.tif", path "G:/ViFFIdata/170721EuglenaN+N-/170721EuglenaN--7/N--7_00497.tif", path "G:/ViFFIdata/170721EuglenaN+N-/170721EuglenaN--7/N--7_00498.tif", path "G:/ViFFIdata/170721EuglenaN+N-/170721EuglenaN--7/N--7_00499.tif", path "G:/ViFFIdata/170721EuglenaN+N-/170721EuglenaN--7/N--7_00500.tif", path "G:/ViFFIdata/170721EuglenaN+N-/170721EuglenaN--7/N--7_00501.tif", path "G:/ViFFIdata/170721EuglenaN+N-/170721EuglenaN--7/N--7_00502.tif", path "G:/ViFFIdata/170721EuglenaN+N-/170721EuglenaN--7/N--7_00503.tif", path "G:/ViFFIdata/170721EuglenaN+N-/170721EuglenaN--7/N--7_00504.tif", path "G:/ViFFIdata/170721EuglenaN+N-/170721EuglenaN--7/N--7_00505.tif", path "G:/ViFFIdata/170721EuglenaN+N-/170721EuglenaN--7/N--7_00506.tif", path "G:/ViFFIdata/170721EuglenaN+N-/170721EuglenaN--7/N--7_00507.tif", path "G:/ViFFIdata/170721EuglenaN+N-/170721EuglenaN--7/N--7_00508.tif", path "G:/ViFFIdata/170721EuglenaN+N-/170721EuglenaN--7/N--7_00509.tif", path "G:/ViFFIdata/170721EuglenaN+N-/170721EuglenaN--7/N--7_00510.tif", path "G:/ViFFIdata/170721EuglenaN+N-/170721EuglenaN--7/N--7_00511.tif", path "G:/ViFFIdata/170721EuglenaN+N-/170721EuglenaN--7/N--7_00512.tif", path "G:/ViFFIdata/170721EuglenaN+N-/170721EuglenaN--7/N--7_00513.tif", path "G:/ViFFIdata/170721EuglenaN+N-/170721EuglenaN--7/N--7_00514.tif", path "G:/ViFFIdata/170721EuglenaN+N-/170721EuglenaN--7/N--7_00515.tif", path "G:/ViFFIdata/170721EuglenaN+N-/170721EuglenaN--7/N--7_00516.tif", path "G:/ViFFIdata/170721EuglenaN+N-/170721EuglenaN--7/N--7_00517.tif", path "G:/ViFFIdata/170721EuglenaN+N-/170721EuglenaN--7/N--7_00518.tif", path "G:/ViFFIdata/170721EuglenaN+N-/170721EuglenaN--7/N--7_00519.tif", path "G:/ViFFIdata/170721EuglenaN+N-/170721EuglenaN--7/N--7_00520.tif", path "G:/ViFFIdata/170721EuglenaN+N-/170721EuglenaN--7/N--7_00521.tif", path "G:/ViFFIdata/170721EuglenaN+N-/170721EuglenaN--7/N--7_00522.tif", path "G:/ViFFIdata/170721EuglenaN+N-/170721EuglenaN--7/N--7_00523.tif", path "G:/ViFFIdata/170721EuglenaN+N-/170721EuglenaN--7/N--7_00524.tif", path "G:/ViFFIdata/170721EuglenaN+N-/170721EuglenaN--7/N--7_00525.tif", path "G:/ViFFIdata/170721EuglenaN+N-/170721EuglenaN--7/N--7_00526.tif", path "G:/ViFFIdata/170721EuglenaN+N-/170721EuglenaN--7/N--7_00527.tif", path "G:/ViFFIdata/170721EuglenaN+N-/170721EuglenaN--7/N--7_00528.tif", path "G:/ViFFIdata/170721EuglenaN+N-/170721EuglenaN--7/N--7_00529.tif", path "G:/ViFFIdata/170721EuglenaN+N-/170721EuglenaN--7/N--7_00530.tif", path "G:/ViFFIdata/170721EuglenaN+N-/170721EuglenaN--7/N--7_00531.tif", path "G:/ViFFIdata/170721EuglenaN+N-/170721EuglenaN--7/N--7_00532.tif", path "G:/ViFFIdata/170721EuglenaN+N-/170721EuglenaN--7/N--7_00533.tif", path "G:/ViFFIdata/170721EuglenaN+N-/170721EuglenaN--7/N--7_00534.tif", path "G:/ViFFIdata/170721EuglenaN+N-/170721EuglenaN--7/N--7_00535.tif", path "G:/ViFFIdata/170721EuglenaN+N-/170721EuglenaN--7/N--7_00536.tif", path "G:/ViFFIdata/170721EuglenaN+N-/170721EuglenaN--7/N--7_00537.tif", path "G:/ViFFIdata/170721EuglenaN+N-/170721EuglenaN--7/N--7_00538.tif", path "G:/ViFFIdata/170721EuglenaN+N-/170721EuglenaN--7/N--7_00539.tif", path "G:/ViFFIdata/170721EuglenaN+N-/170721EuglenaN--7/N--7_00540.tif", path "G:/ViFFIdata/170721EuglenaN+N-/170721EuglenaN--7/N--7_00541.tif", path "G:/ViFFIdata/170721EuglenaN+N-/170721EuglenaN--7/N--7_00542.tif", path "G:/ViFFIdata/170721EuglenaN+N-/170721EuglenaN--7/N--7_00543.tif", path "G:/ViFFIdata/170721EuglenaN+N-/170721EuglenaN--7/N--7_00544.tif", path "G:/ViFFIdata/170721EuglenaN+N-/170721EuglenaN--7/N--7_00545.tif", path "G:/ViFFIdata/170721EuglenaN+N-/170721EuglenaN--7/N--7_00546.tif", path "G:/ViFFIdata/170721EuglenaN+N-/170721EuglenaN--7/N--7_00547.tif", path "G:/ViFFIdata/170721EuglenaN+N-/170721EuglenaN--7/N--7_00548.tif", path "G:/ViFFIdata/170721EuglenaN+N-/170721EuglenaN--7/N--7_00549.tif", path "G:/ViFFIdata/170721EuglenaN+N-/170721EuglenaN--7/N--7_00550.tif", path "G:/ViFFIdata/170721EuglenaN+N-/170721EuglenaN--7/N--7_00551.tif", path "G:/ViFFIdata/170721EuglenaN+N-/170721EuglenaN--7/N--7_00552.tif", path "G:/ViFFIdata/170721EuglenaN+N-/170721EuglenaN--7/N--7_00553.tif", path "G:/ViFFIdata/170721EuglenaN+N-/170721EuglenaN--7/N--7_00554.tif", path "G:/ViFFIdata/170721EuglenaN+N-/170721EuglenaN--7/N--7_00555.tif", path "G:/ViFFIdata/170721EuglenaN+N-/170721EuglenaN--7/N--7_00556.tif", path "G:/ViFFIdata/170721EuglenaN+N-/170721EuglenaN--7/N--7_00557.tif", path "G:/ViFFIdata/170721EuglenaN+N-/170721EuglenaN--7/N--7_00558.tif", path "G:/ViFFIdata/170721EuglenaN+N-/170721EuglenaN--7/N--7_00559.tif", path "G:/ViFFIdata/170721EuglenaN+N-/170721EuglenaN--7/N--7_00560.tif", path "G:/ViFFIdata/170721EuglenaN+N-/170721EuglenaN--7/N--7_00561.tif", path "G:/ViFFIdata/170721EuglenaN+N-/170721EuglenaN--7/N--7_00562.tif", path "G:/ViFFIdata/170721EuglenaN+N-/170721EuglenaN--7/N--7_00563.tif", path "G:/ViFFIdata/170721EuglenaN+N-/170721EuglenaN--7/N--7_00564.tif", path "G:/ViFFIdata/170721EuglenaN+N-/170721EuglenaN--7/N--7_00565.tif", path "G:/ViFFIdata/170721EuglenaN+N-/170721EuglenaN--7/N--7_00566.tif", path "G:/ViFFIdata/170721EuglenaN+N-/170721EuglenaN--7/N--7_00567.tif", path "G:/ViFFIdata/170721EuglenaN+N-/170721EuglenaN--7/N--7_00568.tif", path "G:/ViFFIdata/170721EuglenaN+N-/170721EuglenaN--7/N--7_00569.tif", path "G:/ViFFIdata/170721EuglenaN+N-/170721EuglenaN--7/N--7_00570.tif", path "G:/ViFFIdata/170721EuglenaN+N-/170721EuglenaN--7/N--7_00571.tif", path "G:/ViFFIdata/170721EuglenaN+N-/170721EuglenaN--7/N--7_00572.tif", path "G:/ViFFIdata/170721EuglenaN+N-/170721EuglenaN--7/N--7_00573.tif", path "G:/ViFFIdata/170721EuglenaN+N-/170721EuglenaN--7/N--7_00574.tif", path "G:/ViFFIdata/170721EuglenaN+N-/170721EuglenaN--7/N--7_00575.tif", path "G:/ViFFIdata/170721EuglenaN+N-/170721EuglenaN--7/N--7_00576.tif", path "G:/ViFFIdata/170721EuglenaN+N-/170721EuglenaN--7/N--7_00577.tif", path "G:/ViFFIdata/170721EuglenaN+N-/170721EuglenaN--7/N--7_00578.tif", path "G:/ViFFIdata/170721EuglenaN+N-/170721EuglenaN--7/N--7_00579.tif", path "G:/ViFFIdata/170721EuglenaN+N-/170721EuglenaN--7/N--7_00580.tif", path "G:/ViFFIdata/170721EuglenaN+N-/170721EuglenaN--7/N--7_00581.tif", path "G:/ViFFIdata/170721EuglenaN+N-/170721EuglenaN--7/N--7_00582.tif", path "G:/ViFFIdata/170721EuglenaN+N-/170721EuglenaN--7/N--7_00583.tif", path "G:/ViFFIdata/170721EuglenaN+N-/170721EuglenaN--7/N--7_00584.tif", path "G:/ViFFIdata/170721EuglenaN+N-/170721EuglenaN--7/N--7_00585.tif", path "G:/ViFFIdata/170721EuglenaN+N-/170721EuglenaN--7/N--7_00586.tif", path "G:/ViFFIdata/170721EuglenaN+N-/170721EuglenaN--7/N--7_00587.tif", path "G:/ViFFIdata/170721EuglenaN+N-/170721EuglenaN--7/N--7_00588.tif", path "G:/ViFFIdata/170721EuglenaN+N-/170721EuglenaN--7/N--7_00589.tif", path "G:/ViFFIdata/170721EuglenaN+N-/170721EuglenaN--7/N--7_00590.tif", path "G:/ViFFIdata/170721EuglenaN+N-/170721EuglenaN--7/N--7_00591.tif", path "G:/ViFFIdata/170721EuglenaN+N-/170721EuglenaN--7/N--7_00592.tif", path "G:/ViFFIdata/170721EuglenaN+N-/170721EuglenaN--7/N--7_00593.tif", path "G:/ViFFIdata/170721EuglenaN+N-/170721EuglenaN--7/N--7_00594.tif", path "G:/ViFFIdata/170721EuglenaN+N-/170721EuglenaN--7/N--7_00595.tif", path "G:/ViFFIdata/170721EuglenaN+N-/170721EuglenaN--7/N--7_00596.tif", path "G:/ViFFIdata/170721EuglenaN+N-/170721EuglenaN--7/N--7_00597.tif", path "G:/ViFFIdata/170721EuglenaN+N-/170721EuglenaN--7/N--7_00598.tif", path "G:/ViFFIdata/170721EuglenaN+N-/170721EuglenaN--7/N--7_00599.tif", path "G:/ViFFIdata/170721EuglenaN+N-/170721EuglenaN--7/N--7_00600.tif", path "G:/ViFFIdata/170721EuglenaN+N-/170721EuglenaN--7/N--7_00601.tif", path "G:/ViFFIdata/170721EuglenaN+N-/170721EuglenaN--7/N--7_00602.tif", path "G:/ViFFIdata/170721EuglenaN+N-/170721EuglenaN--7/N--7_00603.tif", path "G:/ViFFIdata/170721EuglenaN+N-/170721EuglenaN--7/N--7_00604.tif", path "G:/ViFFIdata/170721EuglenaN+N-/170721EuglenaN--7/N--7_00605.tif", path "G:/ViFFIdata/170721EuglenaN+N-/170721EuglenaN--7/N--7_00606.tif", path "G:/ViFFIdata/170721EuglenaN+N-/170721EuglenaN--7/N--7_00607.tif", path "G:/ViFFIdata/170721EuglenaN+N-/170721EuglenaN--7/N--7_00608.tif", path "G:/ViFFIdata/170721EuglenaN+N-/170721EuglenaN--7/N--7_00609.tif", path "G:/ViFFIdata/170721EuglenaN+N-/170721EuglenaN--7/N--7_00610.tif", path "G:/ViFFIdata/170721EuglenaN+N-/170721EuglenaN--7/N--7_00611.tif", path "G:/ViFFIdata/170721EuglenaN+N-/170721EuglenaN--7/N--7_00612.tif", path "G:/ViFFIdata/170721EuglenaN+N-/170721EuglenaN--7/N--7_00613.tif", path "G:/ViFFIdata/170721EuglenaN+N-/170721EuglenaN--7/N--7_00614.tif", path "G:/ViFFIdata/170721EuglenaN+N-/170721EuglenaN--7/N--7_00615.tif", path "G:/ViFFIdata/170721EuglenaN+N-/170721EuglenaN--7/N--7_00616.tif", path "G:/ViFFIdata/170721EuglenaN+N-/170721EuglenaN--7/N--7_00617.tif", path "G:/ViFFIdata/170721EuglenaN+N-/170721EuglenaN--7/N--7_00618.tif", path "G:/ViFFIdata/170721EuglenaN+N-/170721EuglenaN--7/N--7_00619.tif", path "G:/ViFFIdata/170721EuglenaN+N-/170721EuglenaN--7/N--7_00620.tif", path "G:/ViFFIdata/170721EuglenaN+N-/170721EuglenaN--7/N--7_00621.tif", path "G:/ViFFIdata/170721EuglenaN+N-/170721EuglenaN--7/N--7_00622.tif", path "G:/ViFFIdata/170721EuglenaN+N-/170721EuglenaN--7/N--7_00623.tif", path "G:/ViFFIdata/170721EuglenaN+N-/170721EuglenaN--7/N--7_00624.tif", path "G:/ViFFIdata/170721EuglenaN+N-/170721EuglenaN--7/N--7_00625.tif", path "G:/ViFFIdata/170721EuglenaN+N-/170721EuglenaN--7/N--7_00626.tif", path "G:/ViFFIdata/170721EuglenaN+N-/170721EuglenaN--7/N--7_00627.tif", path "G:/ViFFIdata/170721EuglenaN+N-/170721EuglenaN--7/N--7_00628.tif", path "G:/ViFFIdata/170721EuglenaN+N-/170721EuglenaN--7/N--7_00629.tif", path "G:/ViFFIdata/170721EuglenaN+N-/170721EuglenaN--7/N--7_00630.tif", path "G:/ViFFIdata/170721EuglenaN+N-/170721EuglenaN--7/N--7_00631.tif", path "G:/ViFFIdata/170721EuglenaN+N-/170721EuglenaN--7/N--7_00632.tif", path "G:/ViFFIdata/170721EuglenaN+N-/170721EuglenaN--7/N--7_00633.tif", path "G:/ViFFIdata/170721EuglenaN+N-/170721EuglenaN--7/N--7_00634.tif", path "G:/ViFFIdata/170721EuglenaN+N-/170721EuglenaN--7/N--7_00635.tif", path "G:/ViFFIdata/170721EuglenaN+N-/170721EuglenaN--7/N--7_00636.tif", path "G:/ViFFIdata/170721EuglenaN+N-/170721EuglenaN--7/N--7_00637.tif", path "G:/ViFFIdata/170721EuglenaN+N-/170721EuglenaN--7/N--7_00638.tif", path "G:/ViFFIdata/170721EuglenaN+N-/170721EuglenaN--7/N--7_00639.tif", path "G:/ViFFIdata/170721EuglenaN+N-/170721EuglenaN--7/N--7_00640.tif", path "G:/ViFFIdata/170721EuglenaN+N-/170721EuglenaN--7/N--7_00641.tif", path "G:/ViFFIdata/170721EuglenaN+N-/170721EuglenaN--7/N--7_00642.tif", path "G:/ViFFIdata/170721EuglenaN+N-/170721EuglenaN--7/N--7_00643.tif", path "G:/ViFFIdata/170721EuglenaN+N-/170721EuglenaN--7/N--7_00644.tif", path "G:/ViFFIdata/170721EuglenaN+N-/170721EuglenaN--7/N--7_00645.tif", path "G:/ViFFIdata/170721EuglenaN+N-/170721EuglenaN--7/N--7_00646.tif", path "G:/ViFFIdata/170721EuglenaN+N-/170721EuglenaN--7/N--7_00647.tif", path "G:/ViFFIdata/170721EuglenaN+N-/170721EuglenaN--7/N--7_00648.tif", path "G:/ViFFIdata/170721EuglenaN+N-/170721EuglenaN--7/N--7_00649.tif", path "G:/ViFFIdata/170721EuglenaN+N-/170721EuglenaN--7/N--7_00650.tif", path "G:/ViFFIdata/170721EuglenaN+N-/170721EuglenaN--7/N--7_00651.tif", path "G:/ViFFIdata/170721EuglenaN+N-/170721EuglenaN--7/N--7_00652.tif", path "G:/ViFFIdata/170721EuglenaN+N-/170721EuglenaN--7/N--7_00653.tif", path "G:/ViFFIdata/170721EuglenaN+N-/170721EuglenaN--7/N--7_00654.tif", path "G:/ViFFIdata/170721EuglenaN+N-/170721EuglenaN--7/N--7_00655.tif", path "G:/ViFFIdata/170721EuglenaN+N-/170721EuglenaN--7/N--7_00656.tif", path "G:/ViFFIdata/170721EuglenaN+N-/170721EuglenaN--7/N--7_00657.tif", path "G:/ViFFIdata/170721EuglenaN+N-/170721EuglenaN--7/N--7_00658.tif", path "G:/ViFFIdata/170721EuglenaN+N-/170721EuglenaN--7/N--7_00659.tif", path "G:/ViFFIdata/170721EuglenaN+N-/170721EuglenaN--7/N--7_00660.tif", path "G:/ViFFIdata/170721EuglenaN+N-/170721EuglenaN--7/N--7_00661.tif", path "G:/ViFFIdata/170721EuglenaN+N-/170721EuglenaN--7/N--7_00662.tif", path "G:/ViFFIdata/170721EuglenaN+N-/170721EuglenaN--7/N--7_00663.tif", path "G:/ViFFIdata/170721EuglenaN+N-/170721EuglenaN--7/N--7_00664.tif", path "G:/ViFFIdata/170721EuglenaN+N-/170721EuglenaN--7/N--7_00665.tif", path "G:/ViFFIdata/170721EuglenaN+N-/170721EuglenaN--7/N--7_00666.tif", path "G:/ViFFIdata/170721EuglenaN+N-/170721EuglenaN--7/N--7_00667.tif", path "G:/ViFFIdata/170721EuglenaN+N-/170721EuglenaN--7/N--7_00668.tif", path "G:/ViFFIdata/170721EuglenaN+N-/170721EuglenaN--7/N--7_00669.tif", path "G:/ViFFIdata/170721EuglenaN+N-/170721EuglenaN--7/N--7_00670.tif", path "G:/ViFFIdata/170721EuglenaN+N-/170721EuglenaN--7/N--7_00671.tif", path "G:/ViFFIdata/170721EuglenaN+N-/170721EuglenaN--7/N--7_00672.tif", path "G:/ViFFIdata/170721EuglenaN+N-/170721EuglenaN--7/N--7_00673.tif", path "G:/ViFFIdata/170721EuglenaN+N-/170721EuglenaN--7/N--7_00674.tif", path "G:/ViFFIdata/170721EuglenaN+N-/170721EuglenaN--7/N--7_00675.tif", path "G:/ViFFIdata/170721EuglenaN+N-/170721EuglenaN--7/N--7_00676.tif", path "G:/ViFFIdata/170721EuglenaN+N-/170721EuglenaN--7/N--7_00677.tif", path "G:/ViFFIdata/170721EuglenaN+N-/170721EuglenaN--7/N--7_00678.tif", path "G:/ViFFIdata/170721EuglenaN+N-/170721EuglenaN--7/N--7_00679.tif", path "G:/ViFFIdata/170721EuglenaN+N-/170721EuglenaN--7/N--7_00680.tif", path "G:/ViFFIdata/170721EuglenaN+N-/170721EuglenaN--7/N--7_00681.tif", path "G:/ViFFIdata/170721EuglenaN+N-/170721EuglenaN--7/N--7_00682.tif", path "G:/ViFFIdata/170721EuglenaN+N-/170721EuglenaN--7/N--7_00683.tif", path "G:/ViFFIdata/170721EuglenaN+N-/170721EuglenaN--7/N--7_00684.tif", path "G:/ViFFIdata/170721EuglenaN+N-/170721EuglenaN--7/N--7_00685.tif", path "G:/ViFFIdata/170721EuglenaN+N-/170721EuglenaN--7/N--7_00686.tif", path "G:/ViFFIdata/170721EuglenaN+N-/170721EuglenaN--7/N--7_00687.tif", path "G:/ViFFIdata/170721EuglenaN+N-/170721EuglenaN--7/N--7_00688.tif", path "G:/ViFFIdata/170721EuglenaN+N-/170721EuglenaN--7/N--7_00689.tif", path "G:/ViFFIdata/170721EuglenaN+N-/170721EuglenaN--7/N--7_00690.tif", path "G:/ViFFIdata/170721EuglenaN+N-/170721EuglenaN--7/N--7_00691.tif", path "G:/ViFFIdata/170721EuglenaN+N-/170721EuglenaN--7/N--7_00692.tif", path "G:/ViFFIdata/170721EuglenaN+N-/170721EuglenaN--7/N--7_00693.tif", path "G:/ViFFIdata/170721EuglenaN+N-/170721EuglenaN--7/N--7_00694.tif", path "G:/ViFFIdata/170721EuglenaN+N-/170721EuglenaN--7/N--7_00695.tif", path "G:/ViFFIdata/170721EuglenaN+N-/170721EuglenaN--7/N--7_00696.tif", path "G:/ViFFIdata/170721EuglenaN+N-/170721EuglenaN--7/N--7_00697.tif", path "G:/ViFFIdata/170721EuglenaN+N-/170721EuglenaN--7/N--7_00698.tif", path "G:/ViFFIdata/170721EuglenaN+N-/170721EuglenaN--7/N--7_00699.tif", path "G:/ViFFIdata/170721EuglenaN+N-/170721EuglenaN--7/N--7_00700.tif", path "G:/ViFFIdata/170721EuglenaN+N-/170721EuglenaN--7/N--7_00701.tif", path "G:/ViFFIdata/170721EuglenaN+N-/170721EuglenaN--7/N--7_00702.tif", path "G:/ViFFIdata/170721EuglenaN+N-/170721EuglenaN--7/N--7_00703.tif", path "G:/ViFFIdata/170721EuglenaN+N-/170721EuglenaN--7/N--7_00704.tif", path "G:/ViFFIdata/170721EuglenaN+N-/170721EuglenaN--7/N--7_00705.tif", path "G:/ViFFIdata/170721EuglenaN+N-/170721EuglenaN--7/N--7_00706.tif", path "G:/ViFFIdata/170721EuglenaN+N-/170721EuglenaN--7/N--7_00707.tif", path "G:/ViFFIdata/170721EuglenaN+N-/170721EuglenaN--7/N--7_00708.tif", path "G:/ViFFIdata/170721EuglenaN+N-/170721EuglenaN--7/N--7_00709.tif", path "G:/ViFFIdata/170721EuglenaN+N-/170721EuglenaN--7/N--7_00710.tif", path "G:/ViFFIdata/170721EuglenaN+N-/170721EuglenaN--7/N--7_00711.tif", path "G:/ViFFIdata/170721EuglenaN+N-/170721EuglenaN--7/N--7_00712.tif", path "G:/ViFFIdata/170721EuglenaN+N-/170721EuglenaN--7/N--7_00713.tif", path "G:/ViFFIdata/170721EuglenaN+N-/170721EuglenaN--7/N--7_00714.tif", path "G:/ViFFIdata/170721EuglenaN+N-/170721EuglenaN--7/N--7_00715.tif", path "G:/ViFFIdata/170721EuglenaN+N-/170721EuglenaN--7/N--7_00716.tif", path "G:/ViFFIdata/170721EuglenaN+N-/170721EuglenaN--7/N--7_00717.tif", path "G:/ViFFIdata/170721EuglenaN+N-/170721EuglenaN--7/N--7_00718.tif", path "G:/ViFFIdata/170721EuglenaN+N-/170721EuglenaN--7/N--7_00719.tif", path "G:/ViFFIdata/170721EuglenaN+N-/170721EuglenaN--7/N--7_00720.tif", path "G:/ViFFIdata/170721EuglenaN+N-/170721EuglenaN--7/N--7_00721.tif", path "G:/ViFFIdata/170721EuglenaN+N-/170721EuglenaN--7/N--7_00722.tif", path "G:/ViFFIdata/170721EuglenaN+N-/170721EuglenaN--7/N--7_00723.tif", path "G:/ViFFIdata/170721EuglenaN+N-/170721EuglenaN--7/N--7_00724.tif", path "G:/ViFFIdata/170721EuglenaN+N-/170721EuglenaN--7/N--7_00725.tif", path "G:/ViFFIdata/170721EuglenaN+N-/170721EuglenaN--7/N--7_00726.tif", path "G:/ViFFIdata/170721EuglenaN+N-/170721EuglenaN--7/N--7_00727.tif", path "G:/ViFFIdata/170721EuglenaN+N-/170721EuglenaN--7/N--7_00728.tif", path "G:/ViFFIdata/170721EuglenaN+N-/170721EuglenaN--7/N--7_00729.tif", path "G:/ViFFIdata/170721EuglenaN+N-/170721EuglenaN--7/N--7_00730.tif", path "G:/ViFFIdata/170721EuglenaN+N-/170721EuglenaN--7/N--7_00731.tif", path "G:/ViFFIdata/170721EuglenaN+N-/170721EuglenaN--7/N--7_00732.tif", path "G:/ViFFIdata/170721EuglenaN+N-/170721EuglenaN--7/N--7_00733.tif", path "G:/ViFFIdata/170721EuglenaN+N-/170721EuglenaN--7/N--7_00734.tif", path "G:/ViFFIdata/170721EuglenaN+N-/170721EuglenaN--7/N--7_00735.tif", path "G:/ViFFIdata/170721EuglenaN+N-/170721EuglenaN--7/N--7_00736.tif", path "G:/ViFFIdata/170721EuglenaN+N-/170721EuglenaN--7/N--7_00737.tif", path "G:/ViFFIdata/170721EuglenaN+N-/170721EuglenaN--7/N--7_00738.tif", path "G:/ViFFIdata/170721EuglenaN+N-/170721EuglenaN--7/N--7_00739.tif", path "G:/ViFFIdata/170721EuglenaN+N-/170721EuglenaN--7/N--7_00740.tif", path "G:/ViFFIdata/170721EuglenaN+N-/170721EuglenaN--7/N--7_00741.tif", path "G:/ViFFIdata/170721EuglenaN+N-/170721EuglenaN--7/N--7_00742.tif", path "G:/ViFFIdata/170721EuglenaN+N-/170721EuglenaN--7/N--7_00743.tif", path "G:/ViFFIdata/170721EuglenaN+N-/170721EuglenaN--7/N--7_00744.tif", path "G:/ViFFIdata/170721EuglenaN+N-/170721EuglenaN--7/N--7_00745.tif", path "G:/ViFFIdata/170721EuglenaN+N-/170721EuglenaN--7/N--7_00746.tif", path "G:/ViFFIdata/170721EuglenaN+N-/170721EuglenaN--7/N--7_00747.tif", path "G:/ViFFIdata/170721EuglenaN+N-/170721EuglenaN--7/N--7_00748.tif", path "G:/ViFFIdata/170721EuglenaN+N-/170721EuglenaN--7/N--7_00749.tif", path "G:/ViFFIdata/170721EuglenaN+N-/170721EuglenaN--7/N--7_00750.tif", path "G:/ViFFIdata/170721EuglenaN+N-/170721EuglenaN--7/N--7_00751.tif", path "G:/ViFFIdata/170721EuglenaN+N-/170721EuglenaN--7/N--7_00752.tif", path "G:/ViFFIdata/170721EuglenaN+N-/170721EuglenaN--7/N--7_00753.tif", path "G:/ViFFIdata/170721EuglenaN+N-/170721EuglenaN--7/N--7_00754.tif", path "G:/ViFFIdata/170721EuglenaN+N-/170721EuglenaN--7/N--7_00755.tif", path "G:/ViFFIdata/170721EuglenaN+N-/170721EuglenaN--7/N--7_00756.tif", path "G:/ViFFIdata/170721EuglenaN+N-/170721EuglenaN--7/N--7_00757.tif", path "G:/ViFFIdata/170721EuglenaN+N-/170721EuglenaN--7/N--7_00758.tif", path "G:/ViFFIdata/170721EuglenaN+N-/170721EuglenaN--7/N--7_00759.tif", path "G:/ViFFIdata/170721EuglenaN+N-/170721EuglenaN--7/N--7_00760.tif", path "G:/ViFFIdata/170721EuglenaN+N-/170721EuglenaN--7/N--7_00761.tif", path "G:/ViFFIdata/170721EuglenaN+N-/170721EuglenaN--7/N--7_00762.tif", path "G:/ViFFIdata/170721EuglenaN+N-/170721EuglenaN--7/N--7_00763.tif", path "G:/ViFFIdata/170721EuglenaN+N-/170721EuglenaN--7/N--7_00764.tif", path "G:/ViFFIdata/170721EuglenaN+N-/170721EuglenaN--7/N--7_00765.tif", path "G:/ViFFIdata/170721EuglenaN+N-/170721EuglenaN--7/N--7_00766.tif", path "G:/ViFFIdata/170721EuglenaN+N-/170721EuglenaN--7/N--7_00767.tif", path "G:/ViFFIdata/170721EuglenaN+N-/170721EuglenaN--7/N--7_00768.tif", path "G:/ViFFIdata/170721EuglenaN+N-/170721EuglenaN--7/N--7_00769.tif", path "G:/ViFFIdata/170721EuglenaN+N-/170721EuglenaN--7/N--7_00770.tif", path "G:/ViFFIdata/170721EuglenaN+N-/170721EuglenaN--7/N--7_00771.tif", path "G:/ViFFIdata/170721EuglenaN+N-/170721EuglenaN--7/N--7_00772.tif", path "G:/ViFFIdata/170721EuglenaN+N-/170721EuglenaN--7/N--7_00773.tif", path "G:/ViFFIdata/170721EuglenaN+N-/170721EuglenaN--7/N--7_00774.tif", path "G:/ViFFIdata/170721EuglenaN+N-/170721EuglenaN--7/N--7_00775.tif", path "G:/ViFFIdata/170721EuglenaN+N-/170721EuglenaN--7/N--7_00776.tif", path "G:/ViFFIdata/170721EuglenaN+N-/170721EuglenaN--7/N--7_00777.tif", path "G:/ViFFIdata/170721EuglenaN+N-/170721EuglenaN--7/N--7_00778.tif", path "G:/ViFFIdata/170721EuglenaN+N-/170721EuglenaN--7/N--7_00779.tif", path "G:/ViFFIdata/170721EuglenaN+N-/170721EuglenaN--7/N--7_00780.tif", path "G:/ViFFIdata/170721EuglenaN+N-/170721EuglenaN--7/N--7_00781.tif", path "G:/ViFFIdata/170721EuglenaN+N-/170721EuglenaN--7/N--7_00782.tif", path "G:/ViFFIdata/170721EuglenaN+N-/170721EuglenaN--7/N--7_00783.tif", path "G:/ViFFIdata/170721EuglenaN+N-/170721EuglenaN--7/N--7_00784.tif", path "G:/ViFFIdata/170721EuglenaN+N-/170721EuglenaN--7/N--7_00785.tif", path "G:/ViFFIdata/170721EuglenaN+N-/170721EuglenaN--7/N--7_00786.tif", path "G:/ViFFIdata/170721EuglenaN+N-/170721EuglenaN--7/N--7_00787.tif", path "G:/ViFFIdata/170721EuglenaN+N-/170721EuglenaN--7/N--7_00788.tif", path "G:/ViFFIdata/170721EuglenaN+N-/170721EuglenaN--7/N--7_00789.tif", path "G:/ViFFIdata/170721EuglenaN+N-/170721EuglenaN--7/N--7_00790.tif", path "G:/ViFFIdata/170721EuglenaN+N-/170721EuglenaN--7/N--7_00791.tif", path "G:/ViFFIdata/170721EuglenaN+N-/170721EuglenaN--7/N--7_00792.tif", path "G:/ViFFIdata/170721EuglenaN+N-/170721EuglenaN--7/N--7_00793.tif", path "G:/ViFFIdata/170721EuglenaN+N-/170721EuglenaN--7/N--7_00794.tif", path "G:/ViFFIdata/170721EuglenaN+N-/170721EuglenaN--7/N--7_00795.tif", path "G:/ViFFIdata/170721EuglenaN+N-/170721EuglenaN--7/N--7_00796.tif", path "G:/ViFFIdata/170721EuglenaN+N-/170721EuglenaN--7/N--7_00797.tif", path "G:/ViFFIdata/170721EuglenaN+N-/170721EuglenaN--7/N--7_00798.tif", path "G:/ViFFIdata/170721EuglenaN+N-/170721EuglenaN--7/N--7_00799.tif", path "G:/ViFFIdata/170721EuglenaN+N-/170721EuglenaN--7/N--7_00800.tif", path "G:/ViFFIdata/170721EuglenaN+N-/170721EuglenaN--7/N--7_00801.tif", path "G:/ViFFIdata/170721EuglenaN+N-/170721EuglenaN--7/N--7_00802.tif", path "G:/ViFFIdata/170721EuglenaN+N-/170721EuglenaN--7/N--7_00803.tif", path "G:/ViFFIdata/170721EuglenaN+N-/170721EuglenaN--7/N--7_00804.tif", path "G:/ViFFIdata/170721EuglenaN+N-/170721EuglenaN--7/N--7_00805.tif", path "G:/ViFFIdata/170721EuglenaN+N-/170721EuglenaN--7/N--7_00806.tif", path "G:/ViFFIdata/170721EuglenaN+N-/170721EuglenaN--7/N--7_00807.tif", path "G:/ViFFIdata/170721EuglenaN+N-/170721EuglenaN--7/N--7_00808.tif", path "G:/ViFFIdata/170721EuglenaN+N-/170721EuglenaN--7/N--7_00809.tif", path "G:/ViFFIdata/170721EuglenaN+N-/170721EuglenaN--7/N--7_00810.tif", path "G:/ViFFIdata/170721EuglenaN+N-/170721EuglenaN--7/N--7_00811.tif", path "G:/ViFFIdata/170721EuglenaN+N-/170721EuglenaN--7/N--7_00812.tif", path "G:/ViFFIdata/170721EuglenaN+N-/170721EuglenaN--7/N--7_00813.tif", path "G:/ViFFIdata/170721EuglenaN+N-/170721EuglenaN--7/N--7_00814.tif", path "G:/ViFFIdata/170721EuglenaN+N-/170721EuglenaN--7/N--7_00815.tif", path "G:/ViFFIdata/170721EuglenaN+N-/170721EuglenaN--7/N--7_00816.tif", path "G:/ViFFIdata/170721EuglenaN+N-/170721EuglenaN--7/N--7_00817.tif", path "G:/ViFFIdata/170721EuglenaN+N-/170721EuglenaN--7/N--7_00818.tif", path "G:/ViFFIdata/170721EuglenaN+N-/170721EuglenaN--7/N--7_00819.tif", path "G:/ViFFIdata/170721EuglenaN+N-/170721EuglenaN--7/N--7_00820.tif", path "G:/ViFFIdata/170721EuglenaN+N-/170721EuglenaN--7/N--7_00821.tif", path "G:/ViFFIdata/170721EuglenaN+N-/170721EuglenaN--7/N--7_00822.tif", path "G:/ViFFIdata/170721EuglenaN+N-/170721EuglenaN--7/N--7_00823.tif", path "G:/ViFFIdata/170721EuglenaN+N-/170721EuglenaN--7/N--7_00824.tif", path "G:/ViFFIdata/170721EuglenaN+N-/170721EuglenaN--7/N--7_00825.tif", path "G:/ViFFIdata/170721EuglenaN+N-/170721EuglenaN--7/N--7_00826.tif", path "G:/ViFFIdata/170721EuglenaN+N-/170721EuglenaN--7/N--7_00827.tif", path "G:/ViFFIdata/170721EuglenaN+N-/170721EuglenaN--7/N--7_00828.tif", path "G:/ViFFIdata/170721EuglenaN+N-/170721EuglenaN--7/N--7_00829.tif", path "G:/ViFFIdata/170721EuglenaN+N-/170721EuglenaN--7/N--7_00830.tif", path "G:/ViFFIdata/170721EuglenaN+N-/170721EuglenaN--7/N--7_00831.tif", path "G:/ViFFIdata/170721EuglenaN+N-/170721EuglenaN--7/N--7_00832.tif", path "G:/ViFFIdata/170721EuglenaN+N-/170721EuglenaN--7/N--7_00833.tif", path "G:/ViFFIdata/170721EuglenaN+N-/170721EuglenaN--7/N--7_00834.tif", path "G:/ViFFIdata/170721EuglenaN+N-/170721EuglenaN--7/N--7_00835.tif", path "G:/ViFFIdata/170721EuglenaN+N-/170721EuglenaN--7/N--7_00836.tif", path "G:/ViFFIdata/170721EuglenaN+N-/170721EuglenaN--7/N--7_00837.tif", path "G:/ViFFIdata/170721EuglenaN+N-/170721EuglenaN--7/N--7_00838.tif", path "G:/ViFFIdata/170721EuglenaN+N-/170721EuglenaN--7/N--7_00839.tif", path "G:/ViFFIdata/170721EuglenaN+N-/170721EuglenaN--7/N--7_00840.tif", path "G:/ViFFIdata/170721EuglenaN+N-/170721EuglenaN--7/N--7_00841.tif", path "G:/ViFFIdata/170721EuglenaN+N-/170721EuglenaN--7/N--7_00842.tif", path "G:/ViFFIdata/170721EuglenaN+N-/170721EuglenaN--7/N--7_00843.tif", path "G:/ViFFIdata/170721EuglenaN+N-/170721EuglenaN--7/N--7_00844.tif", path "G:/ViFFIdata/170721EuglenaN+N-/170721EuglenaN--7/N--7_00845.tif", path "G:/ViFFIdata/170721EuglenaN+N-/170721EuglenaN--7/N--7_00846.tif", path "G:/ViFFIdata/170721EuglenaN+N-/170721EuglenaN--7/N--7_00847.tif", path "G:/ViFFIdata/170721EuglenaN+N-/170721EuglenaN--7/N--7_00848.tif", path "G:/ViFFIdata/170721EuglenaN+N-/170721EuglenaN--7/N--7_00849.tif", path "G:/ViFFIdata/170721EuglenaN+N-/170721EuglenaN--7/N--7_00850.tif", path "G:/ViFFIdata/170721EuglenaN+N-/170721EuglenaN--7/N--7_00851.tif", path "G:/ViFFIdata/170721EuglenaN+N-/170721EuglenaN--7/N--7_00852.tif", path "G:/ViFFIdata/170721EuglenaN+N-/170721EuglenaN--7/N--7_00853.tif", path "G:/ViFFIdata/170721EuglenaN+N-/170721EuglenaN--7/N--7_00854.tif", path "G:/ViFFIdata/170721EuglenaN+N-/170721EuglenaN--7/N--7_00855.tif", path "G:/ViFFIdata/170721EuglenaN+N-/170721EuglenaN--7/N--7_00856.tif", path "G:/ViFFIdata/170721EuglenaN+N-/170721EuglenaN--7/N--7_00857.tif", path "G:/ViFFIdata/170721EuglenaN+N-/170721EuglenaN--7/N--7_00858.tif", path "G:/ViFFIdata/170721EuglenaN+N-/170721EuglenaN--7/N--7_00859.tif", path "G:/ViFFIdata/170721EuglenaN+N-/170721EuglenaN--7/N--7_00860.tif", path "G:/ViFFIdata/170721EuglenaN+N-/170721EuglenaN--7/N--7_00861.tif", path "G:/ViFFIdata/170721EuglenaN+N-/170721EuglenaN--7/N--7_00862.tif", path "G:/ViFFIdata/170721EuglenaN+N-/170721EuglenaN--7/N--7_00863.tif", path "G:/ViFFIdata/170721EuglenaN+N-/170721EuglenaN--7/N--7_00864.tif", path "G:/ViFFIdata/170721EuglenaN+N-/170721EuglenaN--7/N--7_00865.tif", path "G:/ViFFIdata/170721EuglenaN+N-/170721EuglenaN--7/N--7_00866.tif", path "G:/ViFFIdata/170721EuglenaN+N-/170721EuglenaN--7/N--7_00867.tif", path "G:/ViFFIdata/170721EuglenaN+N-/170721EuglenaN--7/N--7_00868.tif", path "G:/ViFFIdata/170721EuglenaN+N-/170721EuglenaN--7/N--7_00869.tif", path "G:/ViFFIdata/170721EuglenaN+N-/170721EuglenaN--7/N--7_00870.tif", path "G:/ViFFIdata/170721EuglenaN+N-/170721EuglenaN--7/N--7_00871.tif", path "G:/ViFFIdata/170721EuglenaN+N-/170721EuglenaN--7/N--7_00872.tif", path "G:/ViFFIdata/170721EuglenaN+N-/170721EuglenaN--7/N--7_00873.tif", path "G:/ViFFIdata/170721EuglenaN+N-/170721EuglenaN--7/N--7_00874.tif", path "G:/ViFFIdata/170721EuglenaN+N-/170721EuglenaN--7/N--7_00875.tif", path "G:/ViFFIdata/170721EuglenaN+N-/170721EuglenaN--7/N--7_00876.tif", path "G:/ViFFIdata/170721EuglenaN+N-/170721EuglenaN--7/N--7_00877.tif", path "G:/ViFFIdata/170721EuglenaN+N-/170721EuglenaN--7/N--7_00878.tif", path "G:/ViFFIdata/170721EuglenaN+N-/170721EuglenaN--7/N--7_00879.tif", path "G:/ViFFIdata/170721EuglenaN+N-/170721EuglenaN--7/N--7_00880.tif", path "G:/ViFFIdata/170721EuglenaN+N-/170721EuglenaN--7/N--7_00881.tif", path "G:/ViFFIdata/170721EuglenaN+N-/170721EuglenaN--7/N--7_00882.tif", path "G:/ViFFIdata/170721EuglenaN+N-/170721EuglenaN--7/N--7_00883.tif", path "G:/ViFFIdata/170721EuglenaN+N-/170721EuglenaN--7/N--7_00884.tif", path "G:/ViFFIdata/170721EuglenaN+N-/170721EuglenaN--7/N--7_00885.tif", path "G:/ViFFIdata/170721EuglenaN+N-/170721EuglenaN--7/N--7_00886.tif", path "G:/ViFFIdata/170721EuglenaN+N-/170721EuglenaN--7/N--7_00887.tif", path "G:/ViFFIdata/170721EuglenaN+N-/170721EuglenaN--7/N--7_00888.tif", path "G:/ViFFIdata/170721EuglenaN+N-/170721EuglenaN--7/N--7_00889.tif", path "G:/ViFFIdata/170721EuglenaN+N-/170721EuglenaN--7/N--7_00890.tif", path "G:/ViFFIdata/170721EuglenaN+N-/170721EuglenaN--7/N--7_00891.tif", path "G:/ViFFIdata/170721EuglenaN+N-/170721EuglenaN--7/N--7_00892.tif", path "G:/ViFFIdata/170721EuglenaN+N-/170721EuglenaN--7/N--7_00893.tif", path "G:/ViFFIdata/170721EuglenaN+N-/170721EuglenaN--7/N--7_00894.tif", path "G:/ViFFIdata/170721EuglenaN+N-/170721EuglenaN--7/N--7_00895.tif", path "G:/ViFFIdata/170721EuglenaN+N-/170721EuglenaN--7/N--7_00896.tif", path "G:/ViFFIdata/170721EuglenaN+N-/170721EuglenaN--7/N--7_00897.tif", path "G:/ViFFIdata/170721EuglenaN+N-/170721EuglenaN--7/N--7_00898.tif", path "G:/ViFFIdata/170721EuglenaN+N-/170721EuglenaN--7/N--7_00899.tif", path "G:/ViFFIdata/170721EuglenaN+N-/170721EuglenaN--7/N--7_00900.tif", path "G:/ViFFIdata/170721EuglenaN+N-/170721EuglenaN--7/N--7_00901.tif", path "G:/ViFFIdata/170721EuglenaN+N-/170721EuglenaN--7/N--7_00902.tif", path "G:/ViFFIdata/170721EuglenaN+N-/170721EuglenaN--7/N--7_00903.tif", path "G:/ViFFIdata/170721EuglenaN+N-/170721EuglenaN--7/N--7_00904.tif", path "G:/ViFFIdata/170721EuglenaN+N-/170721EuglenaN--7/N--7_00905.tif", path "G:/ViFFIdata/170721EuglenaN+N-/170721EuglenaN--7/N--7_00906.tif", path "G:/ViFFIdata/170721EuglenaN+N-/170721EuglenaN--7/N--7_00907.tif", path "G:/ViFFIdata/170721EuglenaN+N-/170721EuglenaN--7/N--7_00908.tif", path "G:/ViFFIdata/170721EuglenaN+N-/170721EuglenaN--7/N--7_00909.tif", path "G:/ViFFIdata/170721EuglenaN+N-/170721EuglenaN--7/N--7_00910.tif", path "G:/ViFFIdata/170721EuglenaN+N-/170721EuglenaN--7/N--7_00911.tif", path "G:/ViFFIdata/170721EuglenaN+N-/170721EuglenaN--7/N--7_00912.tif", path "G:/ViFFIdata/170721EuglenaN+N-/170721EuglenaN--7/N--7_00913.tif", path "G:/ViFFIdata/170721EuglenaN+N-/170721EuglenaN--7/N--7_00914.tif", path "G:/ViFFIdata/170721EuglenaN+N-/170721EuglenaN--7/N--7_00915.tif", path "G:/ViFFIdata/170721EuglenaN+N-/170721EuglenaN--7/N--7_00916.tif", path "G:/ViFFIdata/170721EuglenaN+N-/170721EuglenaN--7/N--7_00917.tif", path "G:/ViFFIdata/170721EuglenaN+N-/170721EuglenaN--7/N--7_00918.tif", path "G:/ViFFIdata/170721EuglenaN+N-/170721EuglenaN--7/N--7_00919.tif", path "G:/ViFFIdata/170721EuglenaN+N-/170721EuglenaN--7/N--7_00920.tif", path "G:/ViFFIdata/170721EuglenaN+N-/170721EuglenaN--7/N--7_00921.tif", path "G:/ViFFIdata/170721EuglenaN+N-/170721EuglenaN--7/N--7_00922.tif", path "G:/ViFFIdata/170721EuglenaN+N-/170721EuglenaN--7/N--7_00923.tif", path "G:/ViFFIdata/170721EuglenaN+N-/170721EuglenaN--7/N--7_00924.tif", path "G:/ViFFIdata/170721EuglenaN+N-/170721EuglenaN--7/N--7_00925.tif", path "G:/ViFFIdata/170721EuglenaN+N-/170721EuglenaN--7/N--7_00926.tif", path "G:/ViFFIdata/170721EuglenaN+N-/170721EuglenaN--7/N--7_00927.tif", path "G:/ViFFIdata/170721EuglenaN+N-/170721EuglenaN--7/N--7_00928.tif", path "G:/ViFFIdata/170721EuglenaN+N-/170721EuglenaN--7/N--7_00929.tif", path "G:/ViFFIdata/170721EuglenaN+N-/170721EuglenaN--7/N--7_00930.tif", path "G:/ViFFIdata/170721EuglenaN+N-/170721EuglenaN--7/N--7_00931.tif", path "G:/ViFFIdata/170721EuglenaN+N-/170721EuglenaN--7/N--7_00932.tif", path "G:/ViFFIdata/170721EuglenaN+N-/170721EuglenaN--7/N--7_00933.tif", path "G:/ViFFIdata/170721EuglenaN+N-/170721EuglenaN--7/N--7_00934.tif", path "G:/ViFFIdata/170721EuglenaN+N-/170721EuglenaN--7/N--7_00935.tif", path "G:/ViFFIdata/170721EuglenaN+N-/170721EuglenaN--7/N--7_00936.tif", path "G:/ViFFIdata/170721EuglenaN+N-/170721EuglenaN--7/N--7_00937.tif", path "G:/ViFFIdata/170721EuglenaN+N-/170721EuglenaN--7/N--7_00938.tif", path "G:/ViFFIdata/170721EuglenaN+N-/170721EuglenaN--7/N--7_00939.tif", path "G:/ViFFIdata/170721EuglenaN+N-/170721EuglenaN--7/N--7_00940.tif", path "G:/ViFFIdata/170721EuglenaN+N-/170721EuglenaN--7/N--7_00941.tif", path "G:/ViFFIdata/170721EuglenaN+N-/170721EuglenaN--7/N--7_00942.tif", path "G:/ViFFIdata/170721EuglenaN+N-/170721EuglenaN--7/N--7_00943.tif", path "G:/ViFFIdata/170721EuglenaN+N-/170721EuglenaN--7/N--7_00944.tif", path "G:/ViFFIdata/170721EuglenaN+N-/170721EuglenaN--7/N--7_00945.tif", path "G:/ViFFIdata/170721EuglenaN+N-/170721EuglenaN--7/N--7_00946.tif", path "G:/ViFFIdata/170721EuglenaN+N-/170721EuglenaN--7/N--7_00947.tif", path "G:/ViFFIdata/170721EuglenaN+N-/170721EuglenaN--7/N--7_00948.tif", path "G:/ViFFIdata/170721EuglenaN+N-/170721EuglenaN--7/N--7_00949.tif", path "G:/ViFFIdata/170721EuglenaN+N-/170721EuglenaN--7/N--7_00950.tif", path "G:/ViFFIdata/170721EuglenaN+N-/170721EuglenaN--7/N--7_00951.tif", path "G:/ViFFIdata/170721EuglenaN+N-/170721EuglenaN--7/N--7_00952.tif", path "G:/ViFFIdata/170721EuglenaN+N-/170721EuglenaN--7/N--7_00953.tif", path "G:/ViFFIdata/170721EuglenaN+N-/170721EuglenaN--7/N--7_00954.tif", path "G:/ViFFIdata/170721EuglenaN+N-/170721EuglenaN--7/N--7_00955.tif", path "G:/ViFFIdata/170721EuglenaN+N-/170721EuglenaN--7/N--7_00956.tif", path "G:/ViFFIdata/170721EuglenaN+N-/170721EuglenaN--7/N--7_00957.tif", path "G:/ViFFIdata/170721EuglenaN+N-/170721EuglenaN--7/N--7_00958.tif", path "G:/ViFFIdata/170721EuglenaN+N-/170721EuglenaN--7/N--7_00959.tif", path "G:/ViFFIdata/170721EuglenaN+N-/170721EuglenaN--7/N--7_00960.tif", path "G:/ViFFIdata/170721EuglenaN+N-/170721EuglenaN--7/N--7_00961.tif", path "G:/ViFFIdata/170721EuglenaN+N-/170721EuglenaN--7/N--7_00962.tif", path "G:/ViFFIdata/170721EuglenaN+N-/170721EuglenaN--7/N--7_00963.tif", path "G:/ViFFIdata/170721EuglenaN+N-/170721EuglenaN--7/N--7_00964.tif", path "G:/ViFFIdata/170721EuglenaN+N-/170721EuglenaN--7/N--7_00965.tif", path "G:/ViFFIdata/170721EuglenaN+N-/170721EuglenaN--7/N--7_00966.tif", path "G:/ViFFIdata/170721EuglenaN+N-/170721EuglenaN--7/N--7_00967.tif", path "G:/ViFFIdata/170721EuglenaN+N-/170721EuglenaN--7/N--7_00968.tif", path "G:/ViFFIdata/170721EuglenaN+N-/170721EuglenaN--7/N--7_00969.tif", path "G:/ViFFIdata/170721EuglenaN+N-/170721EuglenaN--7/N--7_00970.tif", path "G:/ViFFIdata/170721EuglenaN+N-/170721EuglenaN--7/N--7_00971.tif", path "G:/ViFFIdata/170721EuglenaN+N-/170721EuglenaN--7/N--7_00972.tif", path "G:/ViFFIdata/170721EuglenaN+N-/170721EuglenaN--7/N--7_00973.tif", path "G:/ViFFIdata/170721EuglenaN+N-/170721EuglenaN--7/N--7_00974.tif", path "G:/ViFFIdata/170721EuglenaN+N-/170721EuglenaN--7/N--7_00975.tif", path "G:/ViFFIdata/170721EuglenaN+N-/170721EuglenaN--7/N--7_00976.tif", path "G:/ViFFIdata/170721EuglenaN+N-/170721EuglenaN--7/N--7_00977.tif", path "G:/ViFFIdata/170721EuglenaN+N-/170721EuglenaN--7/N--7_00978.tif", path "G:/ViFFIdata/170721EuglenaN+N-/170721EuglenaN--7/N--7_00979.tif", path "G:/ViFFIdata/170721EuglenaN+N-/170721EuglenaN--7/N--7_00980.tif", path "G:/ViFFIdata/170721EuglenaN+N-/170721EuglenaN--7/N--7_00981.tif", path "G:/ViFFIdata/170721EuglenaN+N-/170721EuglenaN--7/N--7_00982.tif", path "G:/ViFFIdata/170721EuglenaN+N-/170721EuglenaN--7/N--7_00983.tif", path "G:/ViFFIdata/170721EuglenaN+N-/170721EuglenaN--7/N--7_00984.tif", path "G:/ViFFIdata/170721EuglenaN+N-/170721EuglenaN--7/N--7_00985.tif", path "G:/ViFFIdata/170721EuglenaN+N-/170721EuglenaN--7/N--7_00986.tif", path "G:/ViFFIdata/170721EuglenaN+N-/170721EuglenaN--7/N--7_00987.tif", path "G:/ViFFIdata/170721EuglenaN+N-/170721EuglenaN--7/N--7_00988.tif", path "G:/ViFFIdata/170721EuglenaN+N-/170721EuglenaN--7/N--7_00989.tif", path "G:/ViFFIdata/170721EuglenaN+N-/170721EuglenaN--7/N--7_00990.tif", path "G:/ViFFIdata/170721EuglenaN+N-/170721EuglenaN--7/N--7_00991.tif", path "G:/ViFFIdata/170721EuglenaN+N-/170721EuglenaN--7/N--7_00992.tif", path "G:/ViFFIdata/170721EuglenaN+N-/170721EuglenaN--7/N--7_00993.tif", path "G:/ViFFIdata/170721EuglenaN+N-/170721EuglenaN--7/N--7_00994.tif", path "G:/ViFFIdata/170721EuglenaN+N-/170721EuglenaN--7/N--7_00995.tif", path "G:/ViFFIdata/170721EuglenaN+N-/170721EuglenaN--7/N--7_00996.tif", path "G:/ViFFIdata/170721EuglenaN+N-/170721EuglenaN--7/N--7_00997.tif", path "G:/ViFFIdata/170721EuglenaN+N-/170721EuglenaN--7/N--7_00998.tif", path "G:/ViFFIdata/170721EuglenaN+N-/170721EuglenaN--7/N--7_00999.tif", path "G:/ViFFIdata/170721EuglenaN+N-/170721EuglenaN--7/N--7_01000.tif"], 1 "section unit":i32=3000, 3 "input array":u16[][][](array[numeric]), 5 "Array":dbl[](array[numeric])=[0.3, 0.6], 9 "partial select":bool=TRUE, 11 "length":i32=1000, 12 "save":bool, 14 "file idx":i32) -> (4 "created bg image":u16[][](array[numeric]), 10 "num of files":i32=1000, 15 "Waveform Graph":dbl[](graph)=[237.0, 239.0, 240.0, 240.0, 241.0, 241.0, 241.0, 241.0, 241.0, 241.0, 242.0, 242.0, 242.0, 242.0, 242.0, 242.0, 242.0, 242.0, 243.0, 243.0, 243.0, 243.0, 243.0, 243.0, 244.0, 244.0, 244.0, 244.0, 244.0, 244.0, 244.0, 244.0, 244.0, 245.0, 245.0, 245.0, 245.0, 245.0, 245.0, 245.0, 245.0, 245.0, 245.0, 245.0, 245.0, 245.0, 245.0, 245.0, 245.0, 246.0, 246.0, 246.0, 246.0, 246.0, 246.0, 246.0, 246.0, 246.0, 246.0, 246.0, 246.0, 246.0, 246.0, 246.0, 247.0, 247.0, 247.0, 247.0, 247.0, 247.0, 247.0, 247.0, 247.0, 247.0, 247.0, 247.0, 247.0, 247.0, 247.0, 247.0, 247.0, 247.0, 247.0, 247.0, 247.0, 247.0, 247.0, 247.0, 248.0, 248.0, 248.0, 248.0, 248.0, 248.0, 248.0, 248.0, 248.0, 248.0, 248.0, 248.0, 248.0, 248.0, 248.0, 248.0, 248.0, 248.0, 248.0, 248.0, 248.0, 248.0, 249.0, 249.0, 249.0, 249.0, 249.0, 249.0, 249.0, 249.0, 249.0, 249.0, 249.0, 250.0, 250.0, 250.0, 250.0, 250.0, 250.0, 250.0, 250.0, 250.0, 250.0, 250.0, 250.0, 250.0, 250.0, 250.0, 250.0, 250.0, 250.0, 250.0, 250.0, 250.0, 250.0, 250.0, 250.0, 250.0, 250.0, 250.0, 250.0, 250.0, 250.0, 250.0, 250.0, 250.0, 250.0, 251.0, 251.0, 251.0, 251.0, 251.0, 251.0, 251.0, 251.0, 251.0, 251.0, 251.0, 251.0, 251.0, 251.0, 251.0, 251.0, 251.0, 251.0, 251.0, 251.0, 251.0, 251.0, 251.0, 251.0, 251.0, 251.0, 252.0, 252.0, 252.0, 252.0, 252.0, 252.0, 252.0, 252.0, 252.0, 252.0, 252.0, 252.0, 252.0, 252.0, 253.0, 253.0, 253.0, 253.0, 253.0, 253.0, 253.0, 253.0, 253.0, 253.0, 253.0, 253.0, 253.0, 253.0, 253.0, 253.0, 253.0, 253.0, 253.0, 253.0, 253.0, 254.0, 254.0, 254.0, 254.0, 254.0, 254.0, 254.0, 254.0, 254.0, 254.0, 254.0, 254.0, 254.0, 254.0, 254.0, 254.0, 254.0, 254.0, 254.0, 254.0, 254.0, 254.0, 254.0, 254.0, 254.0, 254.0, 254.0, 254.0, 254.0, 254.0, 255.0, 255.0, 255.0, 255.0, 255.0, 255.0, 255.0, 255.0, 255.0, 255.0, 255.0, 255.0, 255.0, 255.0, 255.0, 255.0, 255.0, 255.0, 255.0, 255.0, 255.0, 255.0, 255.0, 255.0, 255.0, 255.0, 255.0, 255.0, 255.0, 255.0, 255.0, 255.0, 255.0, 256.0, 256.0, 256.0, 256.0, 256.0, 256.0, 256.0, 256.0, 256.0, 256.0, 256.0, 256.0, 257.0, 257.0, 257.0, 257.0, 257.0, 257.0, 257.0, 257.0, 257.0, 257.0, 257.0, 257.0, 257.0, 257.0, 257.0, 257.0, 257.0, 257.0, 257.0, 257.0, 257.0, 257.0, 257.0, 257.0, 257.0, 257.0, 258.0, 258.0, 258.0, 258.0, 258.0, 258.0, 258.0, 258.0, 258.0, 258.0, 258.0, 258.0, 258.0, 258.0, 258.0, 258.0, 258.0, 258.0, 258.0, 258.0, 258.0, 258.0, 258.0, 258.0, 258.0, 258.0, 259.0, 259.0, 259.0, 259.0, 259.0, 259.0, 259.0, 259.0, 259.0, 259.0, 259.0, 259.0, 259.0, 259.0, 259.0, 259.0, 259.0, 260.0, 260.0, 260.0, 260.0, 260.0, 260.0, 260.0, 260.0, 260.0, 260.0, 260.0, 260.0, 260.0, 260.0, 260.0, 261.0, 261.0, 261.0, 261.0, 261.0, 261.0, 261.0, 261.0, 261.0, 261.0, 261.0, 261.0, 261.0, 261.0, 261.0, 261.0, 261.0, 261.0, 261.0, 261.0, 261.0, 261.0, 261.0, 262.0, 262.0, 262.0, 262.0, 262.0, 262.0, 262.0, 262.0, 262.0, 262.0, 262.0, 262.0, 262.0, 262.0, 262.0, 262.0, 262.0, 262.0, 263.0, 263.0, 263.0, 263.0, 263.0, 263.0, 263.0, 263.0, 263.0, 263.0, 263.0, 263.0, 263.0, 263.0, 264.0, 264.0, 264.0, 264.0, 264.0, 264.0, 264.0, 264.0, 264.0, 264.0, 264.0, 264.0, 264.0, 264.0, 264.0, 264.0, 264.0, 265.0, 265.0, 265.0, 265.0, 265.0, 265.0, 265.0, 265.0, 265.0, 265.0, 265.0, 265.0, 266.0, 266.0, 266.0, 266.0, 266.0, 266.0, 266.0, 266.0, 266.0, 266.0, 266.0, 266.0, 266.0, 266.0, 267.0, 267.0, 267.0, 267.0, 267.0, 267.0, 267.0, 267.0, 267.0, 267.0, 268.0, 268.0, 268.0, 268.0, 268.0, 268.0, 268.0, 268.0, 269.0, 269.0, 269.0, 269.0, 269.0, 269.0, 269.0, 269.0, 269.0, 269.0, 269.0, 269.0, 270.0, 270.0, 270.0, 270.0, 270.0, 270.0, 270.0, 270.0, 271.0, 271.0, 271.0, 271.0, 271.0, 271.0, 271.0, 271.0, 271.0, 271.0, 272.0, 272.0, 272.0, 272.0, 272.0, 272.0, 272.0, 272.0, 272.0, 272.0, 273.0, 273.0, 273.0, 273.0, 273.0, 273.0, 273.0, 273.0, 273.0, 273.0, 274.0, 274.0, 274.0, 274.0, 274.0, 274.0, 274.0, 274.0, 275.0, 275.0, 275.0, 276.0, 276.0, 276.0, 277.0, 277.0, 277.0, 277.0, 277.0, 277.0, 278.0, 278.0, 278.0, 278.0, 279.0, 279.0, 279.0, 279.0, 279.0, 280.0, 280.0, 280.0, 280.0, 280.0, 280.0, 281.0, 281.0, 281.0, 281.0, 281.0, 281.0, 282.0, 282.0, 282.0, 282.0, 282.0, 282.0, 282.0, 283.0, 283.0, 283.0, 284.0, 284.0, 285.0, 285.0, 285.0, 285.0, 286.0, 286.0, 286.0, 287.0, 287.0, 287.0, 288.0, 288.0, 288.0, 289.0, 289.0, 290.0, 290.0, 290.0, 290.0, 290.0, 291.0, 291.0, 291.0, 291.0, 292.0, 292.0, 293.0, 294.0, 294.0, 294.0, 295.0, 295.0, 296.0, 296.0, 297.0, 297.0, 298.0, 298.0, 299.0, 299.0, 299.0, 299.0, 302.0, 302.0, 302.0, 303.0, 303.0, 303.0, 304.0, 305.0, 305.0, 305.0, 305.0, 305.0, 306.0, 307.0, 308.0, 308.0, 308.0, 310.0, 313.0, 314.0, 315.0, 316.0, 327.0, 327.0, 328.0, 328.0, 329.0, 334.0, 337.0, 338.0, 338.0, 338.0, 339.0, 339.0, 341.0, 341.0, 342.0, 342.0, 345.0, 345.0, 347.0, 350.0, 351.0, 352.0, 352.0, 357.0, 359.0, 359.0, 360.0, 361.0, 363.0, 363.0, 364.0, 364.0, 374.0, 375.0, 380.0, 380.0, 381.0, 382.0, 384.0, 390.0, 392.0, 392.0, 393.0, 394.0, 394.0, 395.0, 398.0, 399.0, 401.0, 405.0, 406.0, 410.0, 411.0, 419.0, 421.0, 423.0, 426.0, 429.0, 442.0, 447.0, 458.0, 462.0, 467.0, 470.0, 472.0, 478.0, 479.0, 482.0, 495.0, 510.0, 511.0, 512.0, 518.0, 523.0, 538.0, 538.0, 540.0, 563.0, 564.0, 569.0, 574.0, 579.0, 595.0, 608.0, 612.0, 620.0, 628.0, 633.0, 646.0, 670.0, 692.0, 758.0, 759.0, 787.0, 789.0, 832.0, 837.0, 843.0, 849.0, 852.0, 869.0, 919.0, 939.0, 1044.0, 1058.0, 1089.0, 1132.0, 1133.0, 1168.0, 1187.0, 1234.0, 1291.0, 1332.0, 1346.0, 1359.0, 1360.0, 1373.0, 1395.0, 1532.0, 1577.0, 1887.0, 1913.0, 1921.0, 2030.0, 2063.0, 2104.0, 2172.0, 2175.0, 2252.0, 2275.0, 2359.0, 2371.0, 2732.0, 2743.0, 2857.0, 2943.0, 3011.0, 3085.0, 3221.0, 3250.0, 3260.0, 3270.0, 3582.0, 3621.0, 3764.0, 3803.0, 4309.0, 4410.0, 4638.0, 4819.0, 4920.0, 4992.0, 5130.0, 5147.0, 5331.0, 5349.0, 5813.0, 5816.0, 6009.0, 6013.0, 6037.0, 6039.0, 6104.0, 6116.0, 6187.0, 6271.0, 6353.0, 6381.0, 6384.0, 6412.0, 6515.0, 6535.0, 6558.0, 6589.0, 6640.0, 6688.0, 6694.0, 6720.0, 6803.0, 6966.0, 6973.0, 7029.0, 7051.0, 7126.0, 7193.0, 7238.0, 7299.0, 7314.0, 7318.0, 7322.0, 7324.0, 7365.0, 7391.0, 7414.0, 7470.0, 7473.0, 7476.0, 7589.0, 7664.0, 7700.0, 7810.0, 7841.0, 7953.0, 7973.0, 7980.0, 7986.0, 8022.0, 8057.0, 8134.0, 8155.0, 8217.0, 8246.0, 8248.0, 8293.0, 8378.0, 8382.0, 8391.0, 8405.0, 8407.0, 8442.0, 8445.0, 8517.0, 8524.0, 8545.0, 8581.0, 8587.0, 8618.0, 8647.0, 8651.0, 8667.0, 8696.0, 8765.0, 8821.0, 8830.0, 8837.0, 8864.0, 8865.0, 8934.0, 8951.0, 8993.0, 9010.0, 9014.0, 9055.0, 9056.0, 9096.0, 9144.0, 9224.0, 9228.0, 9252.0, 9309.0, 9312.0, 9330.0, 9435.0, 9441.0, 9450.0, 9612.0, 9628.0, 9629.0, 9683.0, 9702.0, 9771.0, 9823.0, 9868.0, 9888.0, 9908.0, 9913.0, 9971.0, 10027.0, 10037.0, 10059.0, 10118.0, 10208.0, 10312.0, 10316.0, 10331.0, 10334.0, 10377.0, 10408.0, 10449.0, 10465.0, 10525.0, 10551.0, 10578.0, 10644.0, 10662.0, 10664.0, 10667.0, 10694.0, 10735.0, 10799.0, 10811.0, 10833.0, 10844.0, 10875.0, 10875.0, 10944.0, 10962.0, 10999.0, 11082.0, 11144.0, 11178.0, 11221.0, 11256.0, 11267.0, 11277.0, 11400.0, 11743.0, 11749.0, 11805.0, 11893.0, 11989.0, 12137.0, 12174.0, 12697.0, 12731.0, 12782.0, 12845.0, 12968.0, 13164.0, 13404.0, 13422.0, 13917.0, 14056.0, 14148.0, 14171.0, 14375.0, 14521.0, 14862.0, 15065.0, 15381.0, 15462.0, 15774.0, 16093.0, 16672.0, 17646.0, 18581.0, 19405.0, 19633.0, 22622.0, 22802.0, 23781.0, 26129.0])   [LabVIEW 2018]
uses:
  <vilib>/Utility/file.llb/Write Delimited Spreadsheet (I64).vi
  <vilib>/vision/NI_Vision_Development_Module.lvlib
panel:
  out "Numeric 2":i32
  out "Numeric":i32
  out "Waveform Graph 3":u16[](graph)
  in  "index (row)":i32
  out "Waveform Graph 2":u16[](graph)
  in  "Size & Order #":T1={"X Size"=3, "Y Size"=3, "Order #"=4}
  in  "Size & Tolerance":T2={"X Size"=3, "Y Size"=3, "% Tolerance"=40}
  out "error out":errorcluster
  out "Intensity Graph":u16[][](graph)
  in  "index":i32
  in  "name or relative path":string="bg.csv"
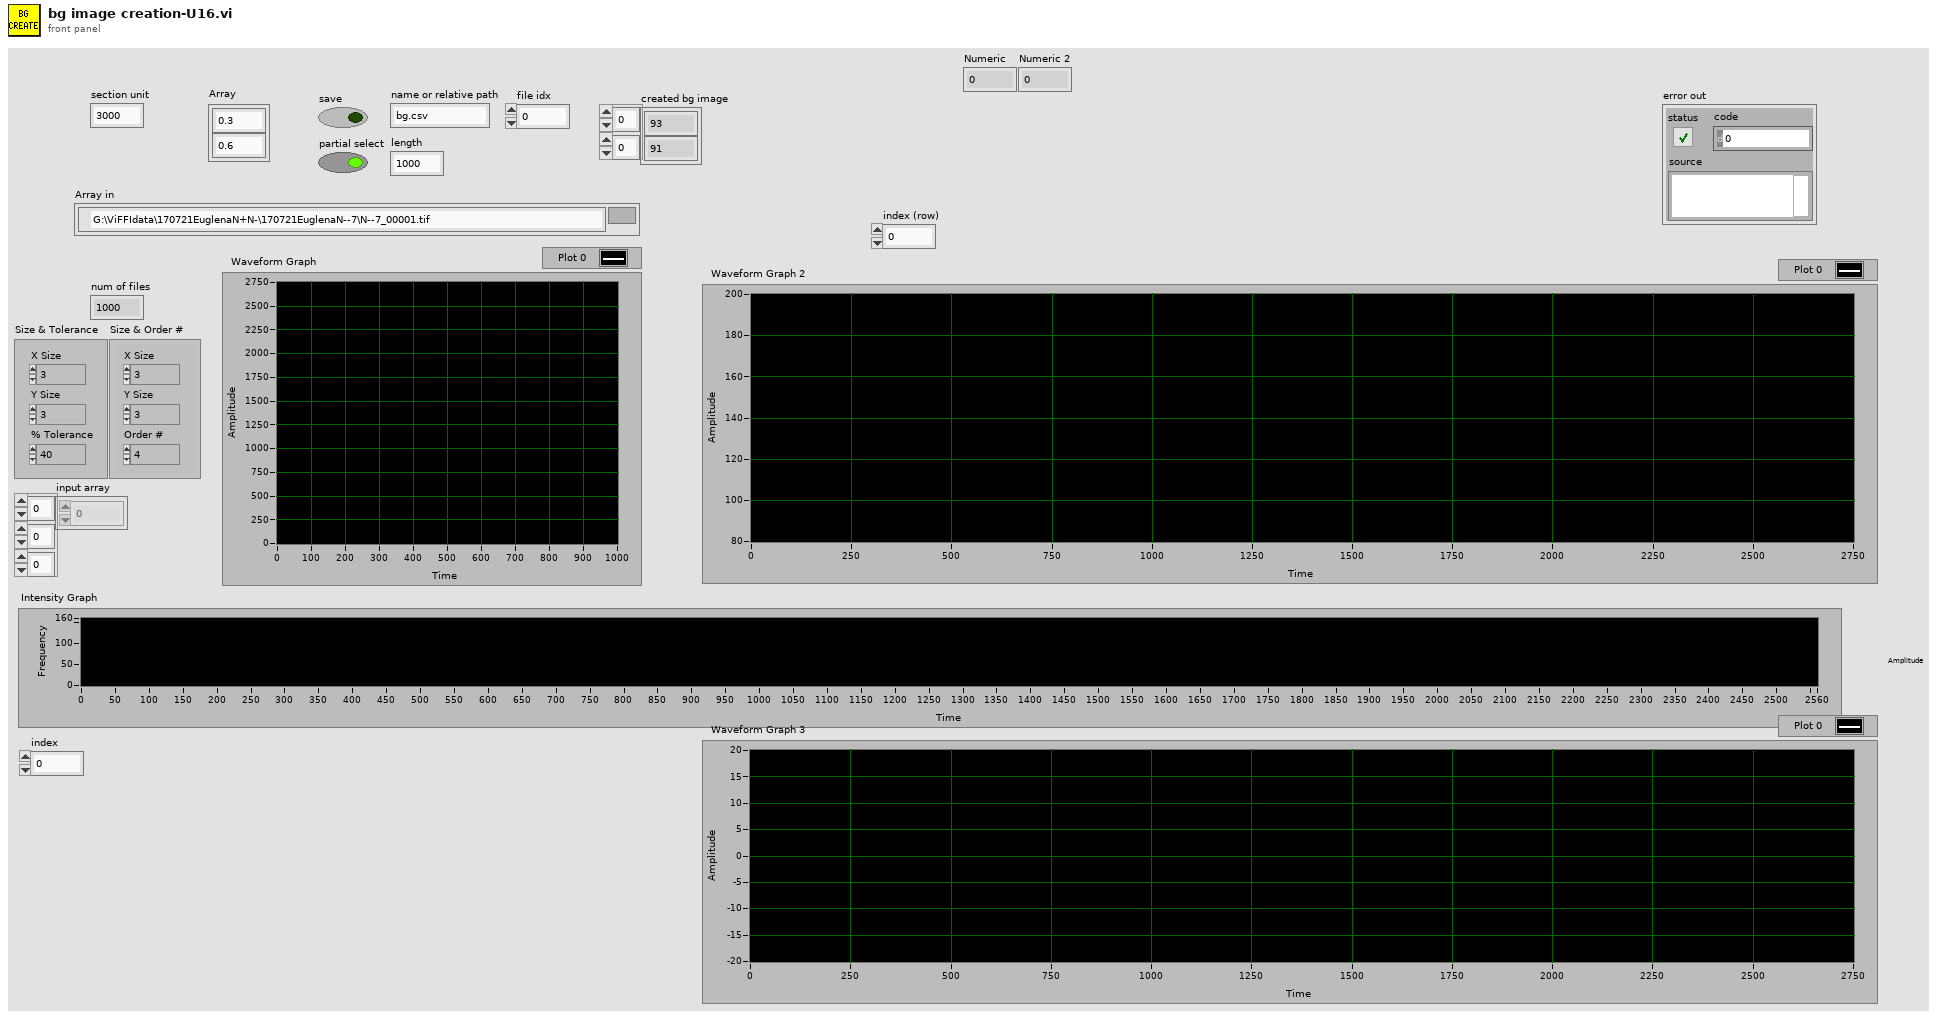
[diagram p1: front panel]
types:
  T1 = cluster{"X Size":i32, "Y Size":i32, "Order #":i32}
  T2 = cluster{"X Size":i32, "Y Size":i32, "% Tolerance":i32}
  T3 = typedef "Image Type" = u32
  T4 = typedef "IMAQ Image.ctl" = refnum<image>
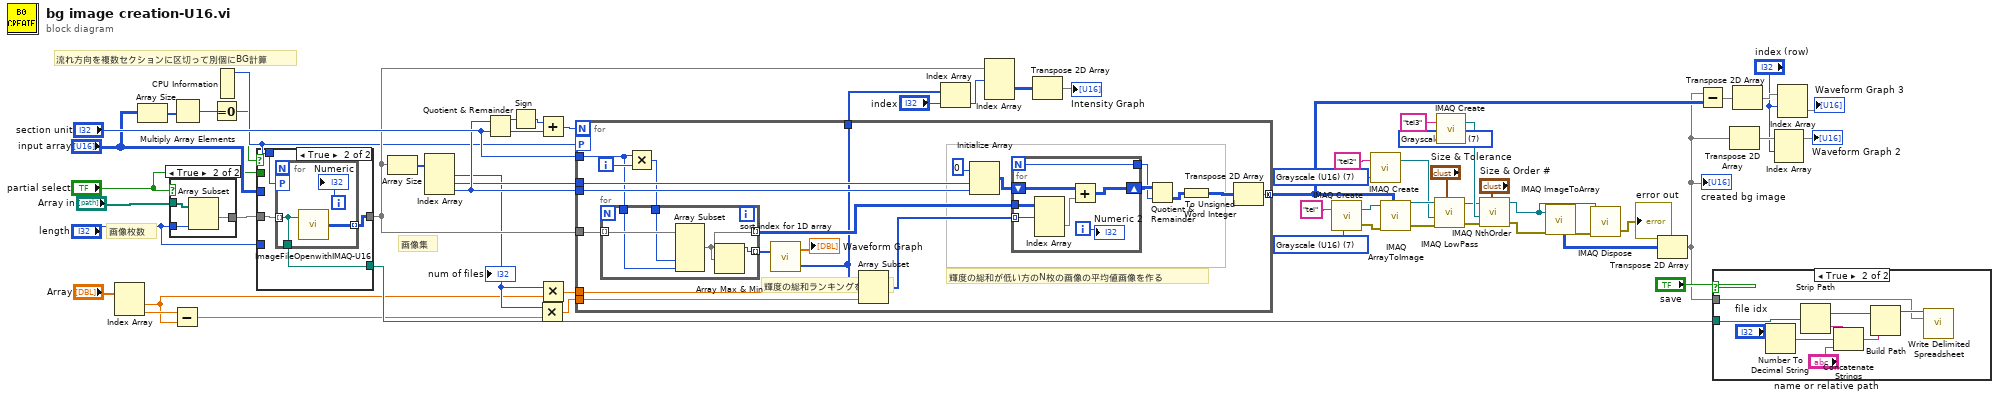
[diagram p0: block diagram]
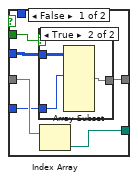
[diagram p2: hidden frame]
diagram:
  w18 = T3 7 items=["Grayscale (U8)", "Grayscale (I16)", "Grayscale (SGL)", "Complex (CSG)", "RGB (U32)", "HSL (U32)", "RGB (U64)", "Grayscale (U16)"] ("Image Type")
  w19 = T3 7 items=["Grayscale (U8)", "Grayscale (I16)", "Grayscale (SGL)", "Complex (CSG)", "RGB (U32)", "HSL (U32)", "RGB (U64)", "Grayscale (U16)"] ("Image Type")
  w20 = T3 7 items=["Grayscale (U8)", "Grayscale (I16)", "Grayscale (SGL)", "Complex (CSG)", "RGB (U32)", "HSL (U32)", "RGB (U64)", "Grayscale (U16)"] ("Image Type")
  # "流れ方向を複数セクションに区切って別個にBG計算"
  # "画像枚数"
  # "画像集"
  n1 = Index Array(array="Array") -> (element #1=w44:dbl, element #2=w46:dbl)  [unwired: 2 in]
  n2 = Array Size(array="input array") -> (size(s)=w7:i32[])
  n3 = case shown="True" "partial select" {
    tunnel: "Array in" -> [w62 w65]
    tunnel: [w62 w64] -> w61
    tunnel: "length" -> [_ w63]
    frame False {
    }
    frame True {
      n4 = Array Subset(array=w65, length=w63) -> (w64:path[])  [unwired: 1 in]
    }
  }
  n5 = Subtract(x=w46, y=w44) -> (x-y=w43:dbl)
  n6 = Multiply Array Elements(1:w7) -> (0:w9:i32)
  n7 = Equal To 0?(x=w9) -> (x = 0?=w6:bool)
  n8 = CPU Information() -> (4:w10:i32)  [unwired: 3 out]
  n9 = case shown="True" w6 {
    tunnel: w61 -> [w71 w79]
    tunnel: [w70 w78] -> w50
    tunnel: [w66 w77] -> w48
    tunnel: w10 -> [_ w76]
    tunnel: "input array" -> [w69 _]
    tunnel: "length" -> [w68 _]
    tunnel: "partial select" -> [w67 _]
    frame False {
      n10 = case shown="True" w67 {
        tunnel: [w72 w75] -> w66
        tunnel: w68 -> [_ w74]
        tunnel: w69 -> [w72 w73]
        frame False {
        }
        frame True {
          n11 = Array Subset(array=w73, length (dim 0)=w74) -> (w75:u16[][][])  [unwired: 5 in]
        }
      }
      n12 = Index Array(array=w71) -> (element=w70:path)  [unwired: 1 in]
    }
    frame True {
      n13 = for {
        tunnel: w79 -> [w81] mode=indexing
        tunnel: [w82] -> w77 mode=indexing
        tunnel: [w81] -> w78
        workers-P: w76 -> [_]
        i -> [w80]
        n14 = call "ImageFileOpenwithIMAQ-U16.vi"("image filepath"=w81) -> ("output array"=w82:u16[][])  [unwired: 1 in]
        "Numeric" <- w80
      }
    }
  }
  n15 = Array Size(array=w48) -> (size(s)=w52:i32[])
  n16 = Index Array(array=w52) -> (element #1=w45:i32, element #2=w53:i32, element #3=w54:i32)  [unwired: 3 in]
  "num of files" <- w45
  n17 = Quotient & Remainder(x=w54, y="section unit") -> (x-y*floor(x/y)=w56:i32, floor(x/y)=w58:i32)
  n18 = Sign(1:w56) -> (0:w57:i32)
  n19 = Multiply(x=w45, y=w43) -> (x*y=w51:dbl)
  n20 = Add(x=w57, y=w58) -> (x+y=w59:i32)
  n21 = Multiply(x=w45, y=w44) -> (x*y=w42:dbl)
  n22 = for {
    N: w59 -> [_]
    tunnel: w48 -> [w98]
    tunnel: [w86] -> w3 mode=concatenating
    tunnel: w51 -> [w92]
    tunnel: w53 -> [w91]
    tunnel: w54 -> [w90]
    tunnel: "section unit" -> [w87]
    tunnel: [w85] -> w49
    tunnel: w42 -> [w84]
    workers-P: w10 -> [_]
    i -> [w89]
    # "輝度の総和ランキングを作る"
    # "輝度の総和が低い方のN枚の画像の平均値画像を作る"
    n23 = Multiply(x=w87, y=w89) -> (x*y=w88:i32)
    n24 = for {
      tunnel: w98 -> [w114] mode=indexing
      tunnel: [w111] -> w102 mode=indexing
      tunnel: [w110] -> w93 mode=indexing
      tunnel: w88 -> [w113]
      tunnel: w87 -> [w112]
      n25 = Array Subset(array=w114, index (col)=w113, length (col)=w112) -> (w110:u16[][])  [unwired: 2 in]
      n26 = Array Max & Min(array=w110) -> (max value=w111:u16)  [unwired: 3 out]
    }
    n27 = call "sort index for 1D array.vi"("Array in"=w102) -> ("index"=w85:i32[], "sorted arrray"=→"Waveform Graph":dbl[])  [unwired: 1 in]
    n28 = Array Subset(array=w85, index=w84, length=w92) -> (w100:i32[])
    n29 = Initialize Array(u32 0 ("element"), w91, w90) -> (w96:u32[][])
    n30 = for {
      N -> [w104]
      tunnel: w100 -> [w108] mode=indexing
      tunnel: w93 -> [w109]
      shift-right: [w106] -> w99
      shift-left: w96 -> [w105]
      tunnel: [w104] -> w94
      i -> [w103]
      n31 = Index Array(array=w109, index (dim 0)=w108) -> (element=w107:u16[][])  [unwired: 2 in]
      n32 = Add(x=w105, y=w107) -> (x+y=w106:u32[][])
      "Numeric 2" <- w103
    }
    n33 = Quotient & Remainder(x=w99, y=w94) -> (floor(x/y)=w95:u32[][])  [unwired: 1 out]
    n34 = To Unsigned Word Integer(number=w95) -> (unsigned 16bit integer=w83:u16[][])
    n35 = Transpose 2D Array(2D array=w83) -> (transposed array=w86:u16[][])
  }
  n36 = Index Array(array=w49, index="index") -> (element=w39:i32)
  n37 = Index Array(array=w48, index (dim 0)=w39) -> (element=w38:u16[][])  [unwired: 2 in]
  n38 = Transpose 2D Array(2D array=w38) -> (transposed array=→"Intensity Graph":u16[][])
  n39 = call "IMAQ Create"("Image Name"="tei", "Image Type"=w18) -> ("New Image"=w35:T4, "error out"=w26:errorcluster)  [unwired: 3 in]
  n40 = call "IMAQ Create"("Image Name"="tei2", "Image Type"=w19) -> ("New Image"=w30:T4)  [unwired: 3 in, 1 out]
  n41 = call "IMAQ ArrayToImage"("Image Pixels (U16)"=w3, "error in (no error)"=w26, "Image"=w35) -> ("error out"=w27:errorcluster, "Image Out"=w34:T4)  [unwired: 7 in]
  n42 = call "IMAQ LowPass"("Image Src"=w34, "Size & Tolerance"="Size & Tolerance", "Image Dst"=w30, "error in (no error)"=w27) -> ("Image Dst Out"=w29:T4, "error out"=w25:errorcluster)  [unwired: 3 in]
  n43 = call "IMAQ Create"("Image Name"="tei3", "Image Type"=w20) -> ("New Image"=w31:T4)  [unwired: 3 in, 1 out]
  n44 = call "IMAQ NthOrder"("Image Src"=w29, "Size & Order #"="Size & Order #", "Image Dst"=w31, "error in (no error)"=w25) -> ("Image Dst Out"=w28:T4, "error out"=w24:errorcluster)  [unwired: 3 in]
  n45 = call "IMAQ ImageToArray"("error in (no error)"=w24, "Image"=w28) -> ("Image Pixels (U16)"=w2:u16[][], "error out"=w23:errorcluster)  [unwired: 2 in, 3 out]
  n46 = call "IMAQ Dispose"("Image"=w28, "error in (no error)"=w23) -> ("error out"=→"error out":errorcluster)  [unwired: 4 in]
  n47 = Transpose 2D Array(2D array=w2) -> (transposed array=w1:u16[][])
  "created bg image" <- w1
  n48 = Subtract(x=w1, y=w3) -> (x-y=w15:u16[][])
  n49 = case shown="True" "save" {
    tunnel: w50 -> [_ w123]
    tunnel: w1 -> [_ w120]
    frame False {
    }
    frame True {
      n50 = Number To Decimal String(number="file idx") -> (decimal integer string=w117:string)  [unwired: 1 in]
      n51 = Strip Path(path=w123) -> (stripped path=w122:path, name=w115:string)
      n52 = Concatenate Strings(w115, w117, "name or relative path") -> (w118:string)
      n53 = Build Path(base path=w122, name or relative path=w118) -> (appended path=w121:path)
      n54 = call-poly <vilib>:"Write Delimited Spreadsheet.vi"("file path (dialog if empty)"=w121, "2D data"=w120) -> ()  [unwired: 12 in, 2 out]
    }
  }
  n55 = Transpose 2D Array(2D array=w1) -> (transposed array=w17:u16[][])
  n56 = Transpose 2D Array(2D array=w15) -> (transposed array=w14:u16[][])
  n57 = Index Array(array=w17, index (row)="index (row)") -> (element=→"Waveform Graph 2":u16[])  [unwired: 1 in]
  n58 = Index Array(array=w14, index (row)="index (row)") -> (element=→"Waveform Graph 3":u16[])  [unwired: 1 in]
